vi "rio 9030 3.vi"() -> ()   [LabVIEW 2015]
uses:
  <vilib>/Platform/TimedLoop/XDataNode/timing_clust.ctl
  <vilib>/Platform/TimedLoop/XDataNode/nitl_modes.ctl
  <vilib>/Platform/TimedLoop/XDataNode/wakeup.ctl
  <vilib>/FPGAPlugInAG/cRIO-9030/niLvFpga_Open_cRIO-9030.vi
  <vilib>/rvi/interface/common/dynamic/niFpgaDynamicAddResources.vi
  <vilib>/FPGAPlugInAG/Dynamic/niLvFpga_Abort_Dynamic.vi
  <vilib>/FPGAPlugInAG/Dynamic/niLvFpga_Run_Dynamic.vi
  rio_Global.vi
  <vilib>/Utility/error.llb/Error Cluster From Error Code.vi
  <vilib>/rvi/errors/niLvFpgaAdjustHostInterfaceError.vi
  <vilib>/Analysis/Matrix/Numeric/Conversions/Array To Matrix - RA2.vi
  <vilib>/Analysis/Matrix/Numeric/Multiply/Multiply - RM,RM.vi
  <vilib>/Analysis/Matrix/Numeric/Add/Add - RM,RM.vi
  <vilib>/Analysis/baseanly.llb/Real Inverse Matrix.vi
  <vilib>/Analysis/Matrix/Numeric/Subtract/Subtract - RM,RM.vi
  <vilib>/Analysis/Matrix/Numeric/Conversions/Array To Matrix - RA.vi
  <vilib>/Analysis/Matrix/Numeric/Multiply/Multiply - R,RM.vi
  <vilib>/Analysis/Matrix/Numeric/Conversions/Matrix To Array - RM.vi
  <vilib>/rvi/interface/nirviOpenFPGA/nirviOpenFPGA.xnode
  FPGA Bitfiles/autonomous_FPGATarget4_fpga1_rudp+OsNkSQ.lvbitx
  samsung/fpga 1.vi
  <vilib>/rvi/interface/nirviMethod/nirviMethod.xnode
  <vilib>/rvi/interface/nirviReadWriteControl/nirviReadWriteControl.xnode
  <vilib>/platform/TimedLoop/XDataNode/XDataNode.xnode
  <vilib>/FPGAPlugInAG/Dynamic/niLvFpga_ReadFifo_Dynamic.vi
  <vilib>/rvi/errors/niLvFpgaMergeErrorWithErrorCode.vi
  <vilib>/Analysis/Matrix/NI_Matrix.lvlib
  <vilib>/Analysis/NI_AALBase.lvlib
  <vilib>/rvi/interface/Simulation/niFpgaSimulationCallBeginRW.vi
  NiFpgaLv.dll
  <vilib>/addons/control/pid/NI_PID_pid.lvlib
  <vilib>/ptbypt/NI_PtbyPt.lvlib
  <vilib>/Platform/TimedLoop/XDataNode/XDNodeRunTimeDep.lvlib
  <vilib>/addons/control/pid/pid.llb/PID (DBL).vi
panel:
  out "vel_ave":dbl
  out "dt vel":dbl
  out "dt":dbl
  in  "GPS on":bool=TRUE
  out "conutpos":i32
  in  "V_PID_gain":dbl[](array[numeric])=[3.0, 10.0, 4.0]
  out "FPGA":refnum<k20>
  in  "GPS Update km/h":dbl=15.0 format="%#_13g"
  out "map name":T1(ring)=enum."KAIST"
  out "con_dt":dbl
  in  "Dial":dbl(knob) min=-360.0 max=360.0 step=5.0 scale=-360.0..360.0
  out "C_yaw_rate":dbl
  in  "speed control":bool
  out "C_MCP":dbl
  out "C_APV":dbl
  out "Ref_VS":dbl
  out "XY Graph":cluster{"Y":dbl[], "Y":dbl[]}[](graph)=[{"Y"=[1.82421875, 1.8301353427767753, 1.835194070339203, 1.8394013252854347, 1.8427635002136231, 1.84528698772192, 1.8469781804084777, 1.8478434708714486, 1.8478892517089844, 1.8471219155192375, 1.84554785490036, 1.8431734624505043, 1.8400051307678222, 1.8360492524504661, 1.8313122200965881, 1.8258004263043404, 1.819520263671875, 1.8124781247973443, 1.8046804022789003, 1.796133488714695, 1.7868437767028809, 1.77681765884161, 1.7660615277290344, 1.7545817759633064, 1.742384796142578, 1.7294769808650017, 1.7158647227287291, 1.701554414331913, 1.686552448272705, 1.6708652171492577, 1.654499113559723, 1.637460530102253, 1.619755859375, 1.6013914939761162, 1.5823738265037537, 1.5627092495560646, 1.5424041557312012, 1.5214649376273155, 1.4998979878425598, 1.4777096989750862, 1.4549064636230469, 1.431494674384594, 1.4074807238578795, 1.3828710046410562, 1.3576719093322753, 1.3318898305296898, 1.3055311608314515, 1.2786022928357124, 1.251109619140625, 1.2230595323443412], "Y"=[0.0, 0.5, 1.0, 1.5, 2.0, 2.5, 3.0, 3.5, 4.0, 4.5, 5.0, 5.5, 6.0, 6.5, 7.0, 7.5, 8.0, 8.5, 9.0, 9.5, 10.0, 10.5, 11.0, 11.5, 12.0, 12.5, 13.0, 13.5, 14.0, 14.5, 15.0, 15.5, 16.0, 16.5, 17.0, 17.5, 18.0, 18.5, 19.0, 19.5, 20.0, 20.5, 21.0, 21.5, 22.0, 22.5, 23.0, 23.5, 24.0, 24.5]}, {"Y"=[-1.22265625, -1.2167396572232247, -1.211680929660797, -1.2074736747145653, -1.2041114997863769, -1.20158801227808, -1.1998968195915223, -1.1990315291285514, -1.1989857482910156, -1.1997530844807625, -1.20132714509964, -1.2037015375494957, -1.2068698692321778, -1.2108257475495339, -1.2155627799034119, -1.2210745736956596, -1.227354736328125, -1.2343968752026557, -1.2421945977210997, -1.250741511285305, -1.2600312232971191, -1.27005734115839, -1.2808134722709656, -1.2922932240366936, -1.304490203857422, -1.3173980191349983, -1.3310102772712709, -1.345320585668087, -1.360322551727295, -1.3760097828507423, -1.392375886440277, -1.409414469897747, -1.427119140625, -1.4454835060238838, -1.4645011734962463, -1.4841657504439354, -1.5044708442687988, -1.5254100623726845, -1.5469770121574402, -1.5691653010249138, -1.5919685363769531, -1.615380325615406, -1.6393942761421205, -1.6640039953589438, -1.6892030906677247, -1.7149851694703102, -1.7413438391685485, -1.7682727071642876, -1.795765380859375, -1.8238154676556588, -1.8524165749549866, -1.8815623101592065, -1.911246280670166, -1.9414620938897134, -1.972203357219696, -2.003463678061962, -2.0352366638183597, -2.0675159218907355, -2.1002950596809384, -2.1335676845908162, -2.167327404022217, -2.2015678253769875, -2.2362825560569766, -2.2714652034640315, -2.307109375, -2.3432086780667305, -2.3797567200660703, -2.4167471083998677, -2.4541734504699706, -2.4920293536782263, -2.530308425426483, -2.5690042731165885, -2.6081105041503907, -2.647620725929737, -2.687528545856476, -2.7278275713324547, -2.7685114097595216, -2.809573668539524, -2.8510079550743104, -2.892807876765728, -2.934967041015625, -2.977479055225849, -3.020337526798248, -3.0635360631346704, -3.107068271636963, -3.150927759706974, -3.1951081347465515, -3.2396030041575434, -3.284405975341797, -3.3295106557011604, -3.3749106526374817, -3.4205995735526087, -3.466571025848389, -3.51281861692667, -3.5593359541893004], "Y"=[0.0, 0.5, 1.0, 1.5, 2.0, 2.5, 3.0, 3.5, 4.0, 4.5, 5.0, 5.5, 6.0, 6.5, 7.0, 7.5, 8.0, 8.5, 9.0, 9.5, 10.0, 10.5, 11.0, 11.5, 12.0, 12.5, 13.0, 13.5, 14.0, 14.5, 15.0, 15.5, 16.0, 16.5, 17.0, 17.5, 18.0, 18.5, 19.0, 19.5, 20.0, 20.5, 21.0, 21.5, 22.0, 22.5, 23.0, 23.5, 24.0, 24.5, 25.0, 25.5, 26.0, 26.5, 27.0, 27.5, 28.0, 28.5, 29.0, 29.5, 30.0, 30.5, 31.0, 31.5, 32.0, 32.5, 33.0, 33.5, 34.0, 34.5, 35.0, 35.5, 36.0, 36.5, 37.0, 37.5, 38.0, 38.5, 39.0, 39.5, 40.0, 40.5, 41.0, 41.5, 42.0, 42.5, 43.0, 43.5, 44.0, 44.5, 45.0, 45.5, 46.0, 46.5, 47.0]}, {"Y"=[-0.94, 0.94, 0.94, -0.94, -0.94], "Y"=[-3.2, -3.2, 1.5, 1.5, -3.2]}, {"Y"=[1.984375, 1.978057861328125, 1.9718017578125, 1.965606689453125, 1.95947265625], "Y"=[0.0, 0.5, 1.0, 1.5, 2.0]}, {"Y"=[-5.28125, -5.267578125, -5.25390625, -5.240234375, -5.2265625], "Y"=[0.0, 0.5, 1.0, 1.5, 2.0]}]
  in  "Manual Steering torque":dbl(slide) min=-0.9 max=0.9 step=0.01 scale=-0.9..0.9
  out "Mobileye_time 50":u32
  out "H_GPS":dbl
  out "vgain":dbl=1.0
  out "vcount":u64=1
  out "hbias":dbl
  out "hcount":u64=1
  out "get heading":bool
  out "get position":bool
  out "heading error":dbl
  out "h_gps":dbl
  out "pos error":dbl
  out "POS init":bool
  out "Heading":dbl
  out "pos":dbl[](array[numeric])
  in  "GPS init":bool=TRUE
  out "pos_gps":dbl[](array[numeric]) format="%#_19f"
  out "dt yaw":dbl
  out "ecef ref":dbl[](array[numeric])
  in  "Velocity input":bool
  in  "Manual Speed":dbl=20.0
  in  "Steer input":bool=TRUE
  out "Run":bool
  out "Auto":bool
  out "E - STOP":bool
  out "Con_time 10":i32
  out "VS_CAN":dbl
  out "CAN_time 10":u32
  out "gps1":refnum<visa-resource-name>
  out "x_view":dbl[](array[numeric])=[0.0, 0.5, 1.0, 1.5, 2.0, 2.5, 3.0, 3.5, 4.0, 4.5, 5.0, 5.5, 6.0, 6.5, 7.0, 7.5, 8.0, 8.5, 9.0, 9.5, 10.0, 10.5, 11.0, 11.5, 12.0, 12.5, 13.0, 13.5, 14.0, 14.5, 15.0, 15.5, 16.0, 16.5, 17.0, 17.5, 18.0, 18.5, 19.0, 19.5, 20.0, 20.5, 21.0, 21.5, 22.0, 22.5, 23.0, 23.5, 24.0, 24.5, 25.0, 25.5, 26.0, 26.5, 27.0, 27.5, 28.0, 28.5, 29.0, 29.5, 30.0, 30.5, 31.0, 31.5, 32.0, 32.5, 33.0, 33.5, 34.0, 34.5, 35.0, 35.5, 36.0, 36.5, 37.0, 37.5, 38.0, 38.5, 39.0, 39.5, 40.0, 40.5, 41.0, 41.5, 42.0, 42.5, 43.0, 43.5, 44.0, 44.5, 45.0, 45.5, 46.0, 46.5, 47.0, 47.5, 48.0, 48.5, 49.0, 49.5, 50.0, 50.5, 51.0, 51.5, 52.0, 52.5, 53.0, 53.5, 54.0, 54.5, 55.0, 55.5, 56.0, 56.5, 57.0, 57.5, 58.0, 58.5, 59.0, 59.5, 60.0, 60.5, 61.0, 61.5, 62.0, 62.5, 63.0, 63.5, 64.0, 64.5, 65.0, 65.5, 66.0, 66.5, 67.0, 67.5, 68.0, 68.5, 69.0, 69.5, 70.0, 70.5, 71.0, 71.5, 72.0, 72.5, 73.0, 73.5, 74.0, 74.5, 75.0, 75.5, 76.0, 76.5, 77.0, 77.5, 78.0, 78.5, 79.0, 79.5, 80.0, 80.5, 81.0, 81.5, 82.0, 82.5, 83.0, 83.5, 84.0, 84.5, 85.0, 85.5, 86.0, 86.5, 87.0, 87.5, 88.0, 88.5, 89.0, 89.5, 90.0, 90.5, 91.0, 91.5, 92.0, 92.5, 93.0, 93.5, 94.0, 94.5, 95.0, 95.5, 96.0, 96.5, 97.0, 97.5, 98.0, 98.5, 99.0, 99.5, 100.0, 100.5, 101.0, 101.5, 102.0, 102.5, 103.0, 103.5, 104.0, 104.5, 105.0, 105.5, 106.0, 106.5, 107.0, 107.5, 108.0, 108.5, 109.0, 109.5, 110.0, 110.5, 111.0, 111.5, 112.0, 112.5, 113.0, 113.5, 114.0, 114.5, 115.0, 115.5, 116.0, 116.5, 117.0, 117.5, 118.0, 118.5, 119.0, 119.5, 120.0, 120.5, 121.0, 121.5, 122.0, 122.5, 123.0, 123.5, 124.0, 124.5, 125.0, 125.5, 126.0, 126.5, 127.0, 127.5, 128.0]
  out "T init":i32
  out "T out":i32
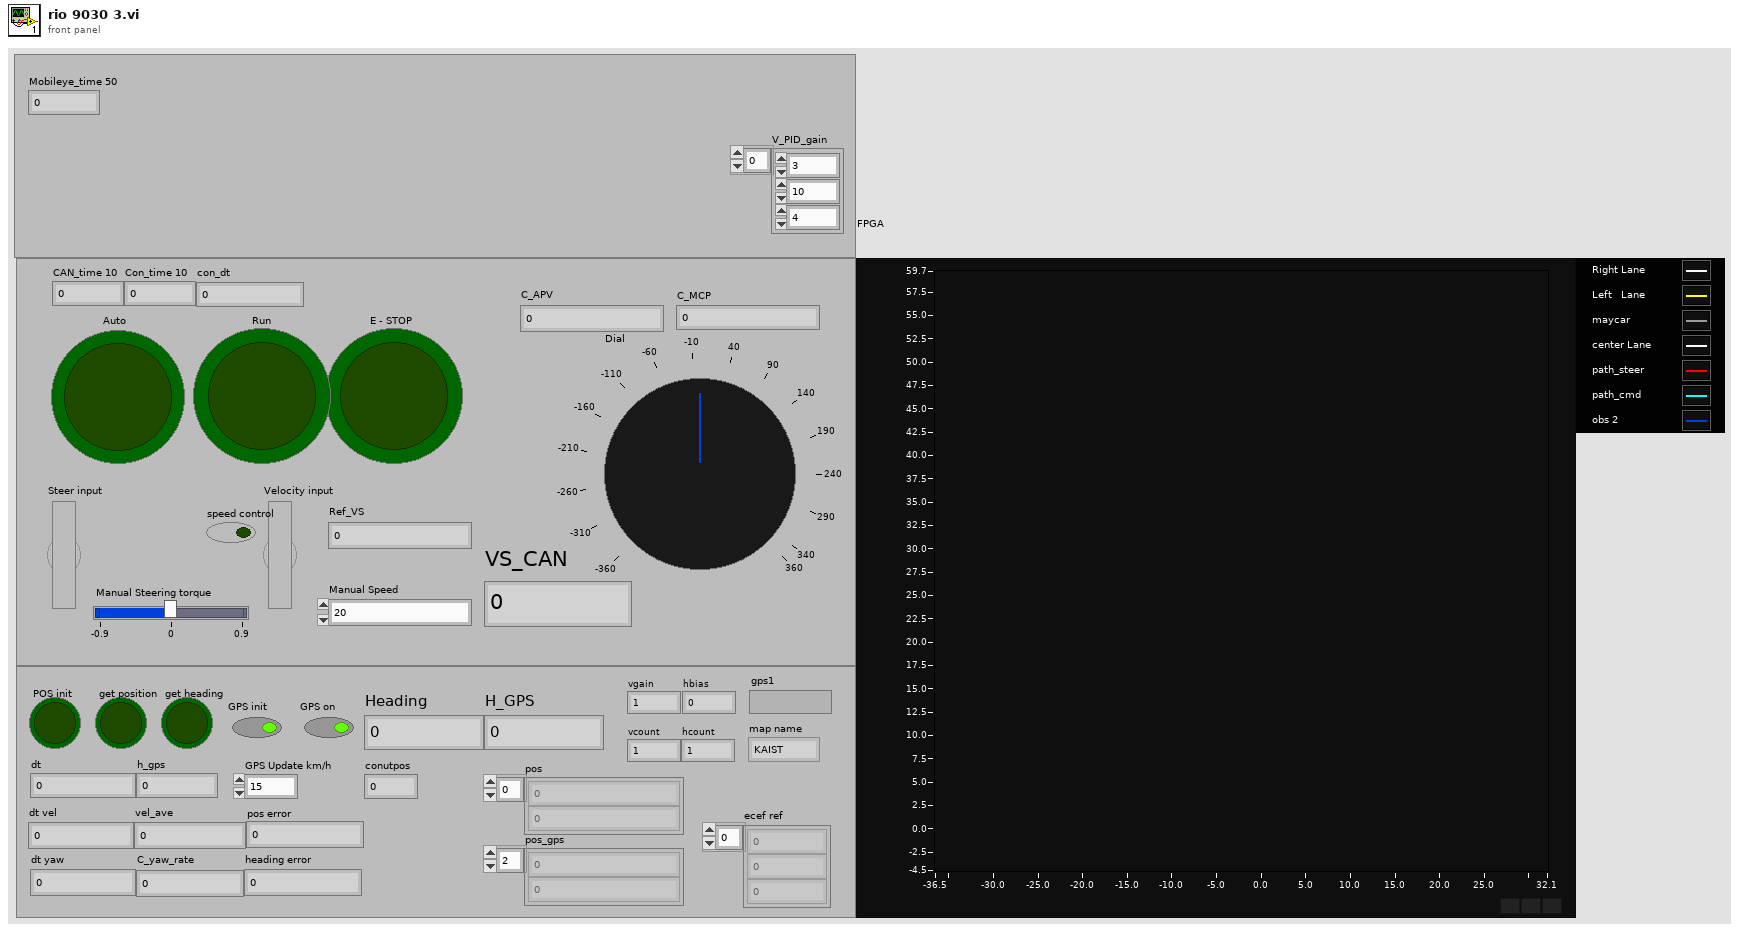
[diagram p1: front panel]
types:
  T1 = enum32{"Namyang", "Hyundai", "KAIST", "Ajou", "Munji", "Airforce", "Car", "KATRI", "Samsung", "Coex", "Gwangnaru", "Inje", "sinjin", "NAVER"}
  T2 = cluster{"identifier":u32, "timestamp":timestamp, "payload":u8[]}
  T3 = cluster{"timestamp high":u32, "timestamp low":u32, "identifier":u32, "type":enum8{"Data Frame", "Remote Frame", "(reserved)", "(reserved) ", "(reserved)  ", "(reserved)   ", "Bus Error", "Transceiver Fault"}, "info A":u8, "info B":u8, "data length":u8, "data":u8[]}
  T4 = cluster{"connection ID":refnum<k16>, "net address":u32, "port":u16}
  T5 = cluster{"hash":i64, "sys time":i64, "size":i32, "data":u8[]}
  T6 = cluster{"hash":i64, "sys time":i64, "time":dbl, "yaw_rate":dbl, "mdps torque":dbl, "mdps str_ang":dbl, "VS_CAN":dbl, "lat_accel":dbl, "mcp":dbl, "accel pedal value":dbl, "tps":dbl, "odometer":dbl, "battery voltage":dbl, "WHL_SPD_RR":dbl, "WHL_SPD_RL":dbl, "WHL_SPD_FR":dbl, "WHL_SPD_FL":dbl}
  T7 = cluster{"proportional gain (Kc)":dbl, "integral time (Ti, min)":dbl, "derivative time (Td, min)":dbl}
  T8 = cluster{"hash":i64, "sys time":i64, "ref_vel":dbl, "ref_steer":dbl, "alert":u8}
  T9 = cluster{"hash":i64, "sys time":i64, "ref_vel":dbl, "ref_steer":dbl}
  T10 = cluster{"hash":i64, "sys time":i64, "Auto":bool, "Run":bool, "Solenoid":bool, "T lim":bool, "brk_enc":u8, "B PWM":u16, "T PWM":u16, "ref_vel":dbl, "ref_bkr_enc":dbl, "ref_apv":dbl, "ref_steer":dbl, "net address":u32}
  T11 = enum32{"Namyang", "Hyundai", "KAIST", "Ajou", "Munji", "Airforce", "Car", "KATRI", "Samsung", "Coex", "Gwangnaru", "Inje", "sinjin"}
  T12 = typedef "XDNodeRunTimeDep.lvlib/timing_clust.ctl" = cluster{"Expected End [f-1]":u64, "Actual End [f-1]":u64, "Finished Late? [f-1]":bool, "Expected End [i-1]":u64, "Actual End [i-1]":u64, "Finished Late? [i-1]":bool, "Expected Start [i]":u64, "Actual Start [i]":u64, "Expected Start [f]":u64, "Actual Start [f]":u64, "Source Name":string, "Structure Name":string, "Period":i64, "Deadline":i64, "Offset":i64, "Start":i64, "Priority":i32, "Timeout":i32, "Mode":T13, "Wakeup Reason":T14, "Error":errorcluster, "Source Type":string, "Secondary Source Type":string, "Global End Time":u64, "Global Start Time":u64, "Frame Duration":u64, "Iteration Duration":u64, "Assigned CPU":i32, "I/O Scan Engine Mode":u32}
  T13 = typedef "XDNodeRunTimeDep.lvlib/nitl_modes.ctl" = enum32{"No Change", "Process missed periods, maintain original phase", "Discard missed periods, maintain original phase", "Process missed periods, ignore original phase", "Discard missed periods, ignore original phase"}
  T14 = typedef "XDNodeRunTimeDep.lvlib/wakeup.ctl" = enum32{"Normal", "Aborted", "Asynchronous wakeup", "Timing source error", "Timed loop error", "Timeout"}
  T15 = cluster{"hash":i64, "sys time":i64, "time":dbl, "x":dbl, "y":dbl, "h":dbl, "numSV":i32, "postype":i32, "lag":i32, "hordev":dbl, "lat":dbl, "lon":dbl, "hgt":dbl, "map_idx":i32}
  T16 = cluster{"output[0]":dbl, "output[1]":dbl, "output[2]":dbl, "output[3]":dbl, "output[4]":dbl, "output[5]":dbl, "output[6]":dbl, "output[7]":dbl, "output[8]":dbl, "output[9]":dbl, "output[10]":dbl, "output[11]":dbl, "output[12]":dbl, "output[13]":dbl, "output[14]":dbl}
  T17 = cluster{"hash":i64, "sys time":i64, "time":dbl, "speed":dbl, "heading":dbl, "lat":dbl, "lon":dbl}
  T18 = cluster{"output[0]":dbl, "output[1]":dbl, "output[2]":dbl, "output[3]":dbl, "output[4]":dbl, "output[5]":dbl, "output[6]":dbl}
  T19 = typedef "NI_Matrix.lvlib/RealMatrix.ctl" = dbl[][]
  T20 = cluster{"hash":i64, "sys time":i64, "dt":dbl, "x":dbl, "y":dbl, "speed":dbl, "heading":dbl, "yaw_rate":dbl}
  T21 = cluster{"Real 2D Array[0]":dbl, "Real 2D Array[1]":dbl, "Real 2D Array[2]":dbl, "Real 2D Array[3]":dbl, "Real 2D Array[4]":dbl}
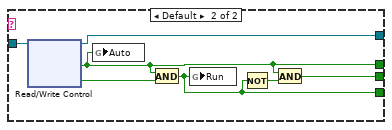
[diagram p3: hidden frame]
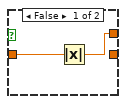
[diagram p7: hidden frame]
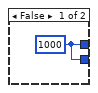
[diagram p8: hidden frame]
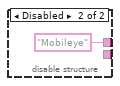
[diagram p9: hidden frame]
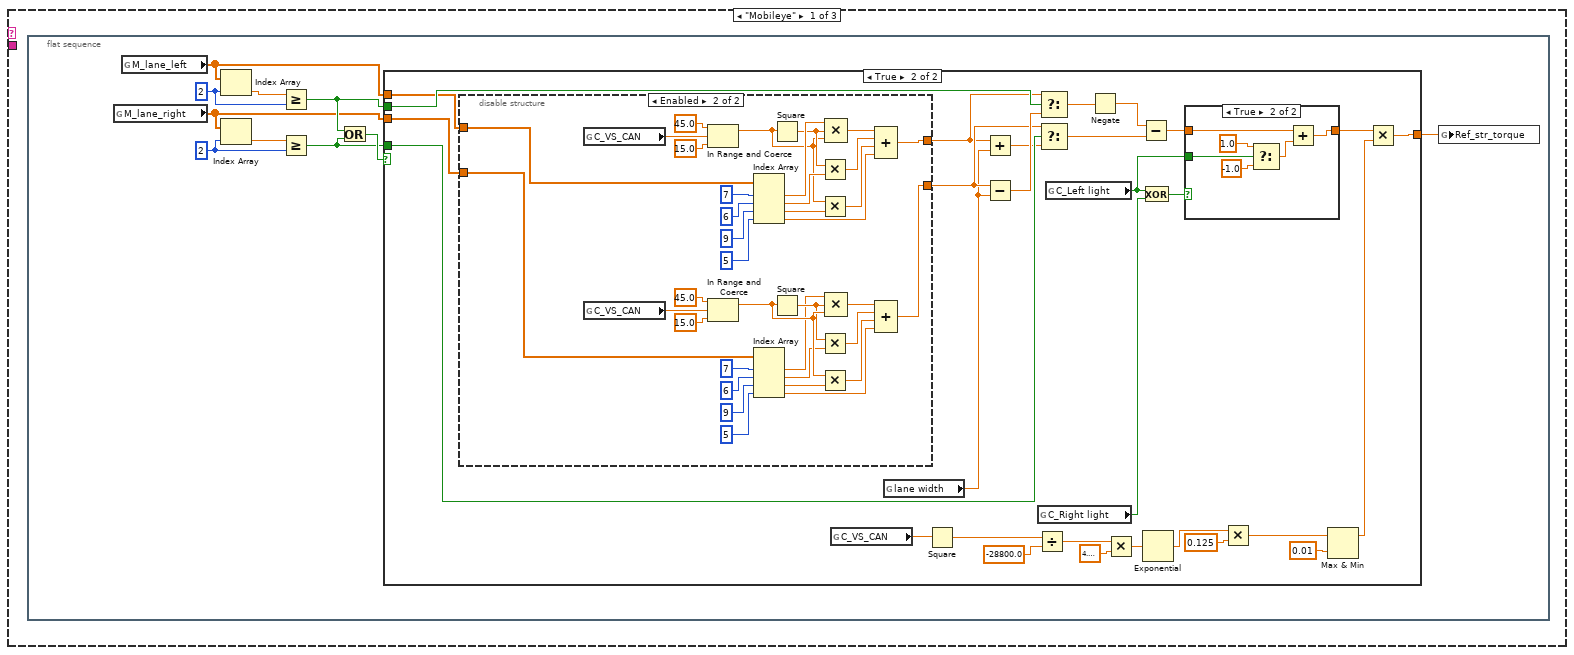
[diagram p10: hidden frame]
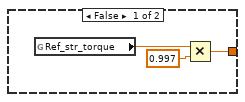
[diagram p11: hidden frame]
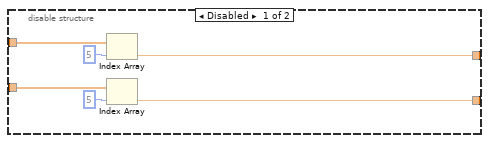
[diagram p12: hidden frame]
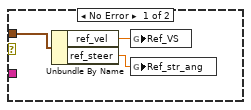
[diagram p14: hidden frame]
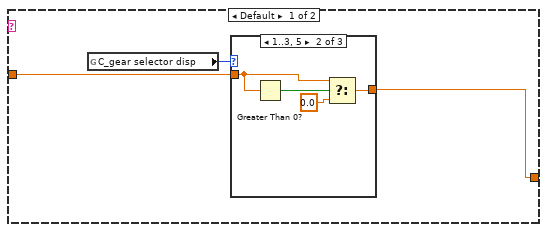
[diagram p17: hidden frame]
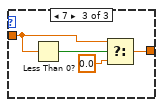
[diagram p19: hidden frame]
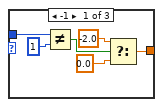
[diagram p20: hidden frame]
diagram:
  n1 = while {
    stop <- FALSE stop-if-true
    n2 = flat-sequence {
      tunnel: [w8] -> w2
      tunnel: w2 -> [w38]
      frame #0 {
        n3 = Wait Until Next ms Multiple(millisecond multiple=u32 10) -> ()  [unwired: 1 out]
      }
      frame #1 {
        n4 = global read "rio_Global.vi" "Car_name"() -> (w5:string)
        n5 = local read "FPGA"() -> (w10:refnum<k20>)
        n6 = case shown="\"Prius\", \"Santafe\"" w5 {
          tunnel: w10 -> [w13 w20]
          tunnel: [_ w18] -> w9
          tunnel: [w13 w16] -> w8
          tunnel: [w12 w15] -> w7
          tunnel: [w11 w14] -> w6
          frame "Prius", "Santafe" {
            n7 = global read "rio_Global.vi" "Auto"() -> (w12:bool)
            n8 = global read "rio_Global.vi" "Run"() -> (w11:bool)
          }
          frame Default {
            n9 = xnode "Read/Write Control"("FPGA VI Reference In"=w20) -> ("FPGA VI Reference Out"=w16:refnum<k20>, "Auto"=w15:bool, "Run"=w19:bool)  [unwired: 1 in, 1 out]
            n10 = global write "rio_Global.vi" "Auto"(w15) -> ()
            n11 = And(x=w15, y=w19) -> (x .and. y?=w14:bool)
            n12 = global write "rio_Global.vi" "Run"(w14) -> ()
            n13 = Not(x=w14) -> (.not. x?=w17:bool)
            n14 = And(x=w15, y=w17) -> (x .and. y?=w18:bool)
          }
        }
        "E - STOP" <- w9
        "Auto" <- w7
        "Run" <- w6
      }
      frame #2 {
        w30 = fxp<+/-,20,5> 0.0 ("Mod3/AO3")
        n15 = global read "rio_Global.vi" "Car_name"() -> (w26:string)
        n16 = global read "rio_Global.vi" "Auto"() -> (w24:bool)
        n17 = case shown="\"Prius\"" w26 {
          tunnel: [_ w42] -> w28
          tunnel: [_ w41] -> w21
          frame Default {
          }
          frame "Prius" {
            n18 = global read "rio_Global.vi" "Shift control"() -> (w43:dbl)
            n19 = global read "rio_Global.vi" "C_VS_CAN"() -> (w45:dbl)
            n20 = Not Equal To 0?(x=w43) -> (x != 0?=w40:bool)
            n21 = Equal To 0?(x=w45) -> (x = 0?=w46:bool)
            n22 = global read "rio_Global.vi" "Auto"() -> (w39:bool)
            n23 = Compound Arithmetic op=AND(w40, w46, w39) -> (w44:bool)
            n24 = case shown="True" w44 {
              selector: w44 -> [_ w47]
              tunnel: w43 -> [_ w48]
              tunnel: [_ w48] -> w42
              tunnel: [_ w47] -> w41
              frame False {
              }
              frame True {
              }
            }
          }
        }
        n25 = global read "rio_Global.vi" "Auto"() -> (w29:bool)
        n26 = And(x="speed control", y=w24) -> (x .and. y?=w23:bool)
        n27 = case shown="True" w23 {
          tunnel: [w56 w69] -> w37
          tunnel: [w56 w68] -> w36
          tunnel: [_ w63] -> w35
          frame False {
            w56 = u16 1000
          }
          frame True {
            n28 = global read "rio_Global.vi" "PWM Brake"() -> (w62:dbl)
            n29 = global read "rio_Global.vi" "PWM GAS"() -> (w71:dbl)
            n30 = Round To Nearest(number=w71) -> (nearest integer value=w66:dbl)
            n31 = Round To Nearest(number=w62) -> (nearest integer value=w61:dbl)
            n32 = global read "rio_Global.vi" "Run"() -> (w59:bool)
            n33 = global read "rio_Global.vi" "Run"() -> (w60:bool)
            n34 = global read "rio_Global.vi" "Solenoid"() -> (w65:bool)
            n35 = Select(t=w66, s=w59, f=1000.0) -> (s? t:f=w64:dbl)
            n36 = Select(t=w61, s=w60, f=1900.0 ("t")) -> (s? t:f=w57:dbl)
            n37 = global read "rio_Global.vi" "Run"() -> (w58:bool)
            n38 = To Unsigned Word Integer(number=w64) -> (unsigned 16bit integer=w69:u16)
            n39 = To Unsigned Word Integer(number=w57) -> (unsigned 16bit integer=w68:u16)
            n40 = Select(t=w65, s=w58, f=w58) -> (s? t:f=w63:bool)
          }
        }
        n41 = case shown="True" w29 {
          tunnel: [_ w50] -> w34
          tunnel: [_ w49] -> w33
          frame False {
          }
          frame True {
            n42 = global read "rio_Global.vi" "steering torque"() -> (w51:dbl)
            n43 = Greater Than 0?(x=w51) -> (x > 0?=w52:bool)
            n44 = case shown="True" w52 {
              tunnel: w51 -> [w54 w55]
              tunnel: [w53 _] -> w50
              tunnel: [_ w55] -> w49
              frame False {
                n45 = Absolute Value(x=w54) -> (abs(x)=w53:dbl)
              }
              frame True {
              }
            }
          }
        }
        n46 = To Fixed-Point(fixed-point type=w30, number=w34) -> (fixed-point=w32:fxp<+/-,20,5>)
        n47 = To Fixed-Point(fixed-point type=w30, number=w33) -> (fixed-point=w31:fxp<+/-,20,5>)
        n48 = To Fixed-Point(fixed-point type=fxp<+/-,20,5> 0.0 ("Mod3/AO3"), number=w28) -> (fixed-point=w22:fxp<+/-,20,5>)
        n49 = xnode "Read/Write Control"("FPGA VI Reference In"=w38, "Solenoid"=w35, "PWM Gas"=w37, "PWM Brake"=w36, "Mod3/AO0"=w32, "Mod3/AO1"=w31, "Mod3/AO3"=w22, "Mod1/DIO3"=w21) -> ()  [unwired: 1 in, 2 out]
      }
    }
  }
  n50 = flat-sequence {
    frame #0 {
      w73 = u16 7668 ("port")
      w82 = u16 7667 ("port")
      n51 = disable-structure shown="Enabled" {
        frame Disabled {
        }
        frame Enabled {
          w90 = "Prius" ("Car_name")
          w96 = 0.0 ("Ref_str_ang")
          w97 = 1000.0 ("PWM GAS")
          w95 = FALSE ("Auto SW")
          n52 = global write "rio_Global.vi" "Shift control"(0.0 ("Shift control")) -> ()
          n53 = global write "rio_Global.vi" "steering torque"(0.0 ("steering")) -> ()
          n54 = global write "rio_Global.vi" "Solenoid"(FALSE ("CAN A 1")) -> ()
          n55 = global write "rio_Global.vi" "Ref_VS"(w96) -> ()
          n56 = global write "rio_Global.vi" "Ref_str_ang"(w96) -> ()
          n57 = global write "rio_Global.vi" "PWM GAS"(w97) -> ()
          n58 = global write "rio_Global.vi" "PWM Brake"(w97) -> ()
          n59 = global write "rio_Global.vi" "Auto"(w95) -> ()
          n60 = global write "rio_Global.vi" "Car_name"(w90) -> ()
          n61 = call "car_spec.vi"("Car_name"=w90) -> ("turn radius"=w94:dbl, "wheel base"=w93:dbl, "ratio"=w92:dbl, "overall width"=w91:dbl)  [unwired: 5 in, 2 out]
          n62 = global write "rio_Global.vi" "Auto SW"(w95) -> ()
          n63 = global write "rio_Global.vi" "ratio"(w92) -> ()
          n64 = global write "rio_Global.vi" "overall width"(w91) -> ()
          n65 = global write "rio_Global.vi" "wheel base"(w93) -> ()
          n66 = global write "rio_Global.vi" "turn radius"(w94) -> ()
        }
      }
      n67 = xnode "Open FPGA VI Reference"() -> ("FPGA VI Reference Out"=w84:refnum<k20>, "error out"=w85:errorcluster)  [unwired: 2 in]
      n68 = global read "rio_Global.vi" "LCM PC"() -> (w77:T4)
      n69 = Decrement(x=w82) -> (x-1=w83:u16)
      n70 = UDP Open(11:w73) -> (port=w75:refnum<k16>)  [unwired: 4 in, 2 out]
      n71 = xnode "Invoke Method"("FPGA VI Reference In"=w84, "error in"=w85) -> ("FPGA VI Reference Out"=w86:refnum<k20>, "error out"=w87:errorcluster)
      n72 = Bundle By Name(cluster=w77, "port"=w73, "connection ID"=w75, "net address"=u32 0) -> (w76:T4)
      n73 = UDP Open(11:w83) -> (port=w80:refnum<k16>)  [unwired: 4 in, 2 out]
      n74 = xnode "Invoke Method"("FPGA VI Reference In"=w86, "error in"=w87, "Wait Until Done (F)"=FALSE) -> ("FPGA VI Reference Out"=→"FPGA":refnum<k20>)  [unwired: 1 out]
      n75 = global read "rio_Global.vi" "LCM"() -> (w78:T4)
      n76 = Bundle By Name(cluster=w78, "port"=w82, "connection ID"=w80, "net address"=u32 4294967295) -> (w79:T4)
      n77 = global write "rio_Global.vi" "LCM PC"(w76) -> ()
      n78 = global write "rio_Global.vi" "LCM"(w79) -> ()
    }
    frame #1 {
      n79 = flat-sequence {
        tunnel: [w102] -> w101
        tunnel: w101 -> [w109]
        frame #0 {
          n80 = local read "FPGA"() -> (w103:refnum<k20>)
          n81 = xnode "Invoke Method"("FPGA VI Reference In"=w103, "Number of Elements"=u32 0, "Timeout (ms)"=0) -> ("FPGA VI Reference Out"=w105:refnum<k20>, "Elements Remaining"=w106:u32)  [unwired: 1 in, 2 out]
          n82 = xnode "Invoke Method"("FPGA VI Reference In"=w105, "Number of Elements"=w106, "Timeout (ms)"=0) -> ("FPGA VI Reference Out"=w102:refnum<k20>)  [unwired: 1 in, 3 out]
        }
        frame #1 {
          n83 = while {
            tunnel: w109 -> [w110]
            stop <- FALSE stop-if-true
            n84 = flat-sequence {
              tunnel: [w113] -> w111
              tunnel: w110 -> [w113]
              tunnel: w111 -> [w120]
              frame #0 {
                n85 = Wait Until Next ms Multiple(millisecond multiple=u32 50) -> (millisecond timer value=w115:u32)
                n86 = feedback #1(w115) -> (w116:u32)
                n87 = feedback-in #1(w115) -> ()
                n88 = Subtract(x=w115, y=w116) -> (x-y=→"Mobileye_time 50":u32)
              }
              frame #1 {
                n89 = while {
                  tunnel: w120 -> [w166]
                  tunnel: [w163] -> w119 mode=indexing
                  stop <- w161 stop-if-true
                  n90 = xnode "Invoke Method"("FPGA VI Reference In"=w166, "Number of Elements"=u32 16, "Timeout (ms)"=0) -> ("FPGA VI Reference Out"=w162:refnum<k20>, "Data"=w163:u8[], "Elements Remaining"=w160:u32)  [unwired: 1 in, 1 out]
                  n91 = Equal To 0?(x=w160) -> (x = 0?=w161:bool)
                  n92 = Quotient & Remainder(x=w160, y=u32 16) -> (x-y*floor(x/y)=w158:u32)  [unwired: 1 out]
                  n93 = case shown="1, Default" w158 {
                    selector: w158 -> [w169 _]
                    tunnel: w162 -> [w168 _]
                    frame 1, Default {
                      n94 = xnode "Invoke Method"("FPGA VI Reference In"=w168, "Number of Elements"=w169, "Timeout (ms)"=0) -> ()  [unwired: 1 in, 4 out]
                    }
                    frame 0 {
                    }
                  }
                }
                n95 = Empty Array?(array=w119) -> (empty?=w118:bool)
                n96 = case shown="False" w118 {
                  tunnel: w119 -> [w122 _]
                  frame False {
                    n97 = flat-sequence {
                      tunnel: w122 -> [w123]
                      tunnel: [w123] -> w121
                      tunnel: w121 -> [w142]
                      frame #0 {
                        n98 = for {
                          tunnel: w123 -> [w133] mode=indexing
                          w136 = 4 ("length")
                          w134 = 8 ("index")
                          n99 = Delete From Array(array=w133, length=w134, index=w134) -> (deleted portion=w124:u8[], array with subset deleted=w135:u8[])
                          n100 = Delete From Array(array=w135, length=w136, index=w136) -> (deleted portion=w140:u8[], array with subset deleted=w137:u8[])
                          n101 = Type Cast(type=u32 0, x=w137) -> (*(type *) &x=w125:u32)
                          n102 = Type Cast(type=u32 0, x=w140) -> (*(type *) &x=w126:u32)
                          n103 = Multiply(x=w126, y=1e-07) -> (x*y=w131:dbl)
                          n104 = To Time Stamp(1:w131) -> (0:w129:timestamp)
                          n105 = Bundle By Name(cluster=T2 {"identifier"=0, "timestamp"=timestamp(0 s since 1904-01-01), "payload"=[]} ("can cluster"), "identifier"=w125, "payload"=w124, "timestamp"=w129) -> (w127:T2)
                          n106 = call "mobileye_decoder.vi"("can cluster"=w127, "name"="Mobileye560") -> ()  [unwired: 10 in]
                        }
                      }
                      frame #1 {
                        n107 = Array Size(array=w142) -> (size(s)=w143:i32[])
                        n108 = Multiply Array Elements(1:w143) -> (0:w152:i32)
                        n109 = Get Date/Time In Seconds() -> (seconds since 1Jan1904=w148:timestamp)
                        n110 = To Double Precision Float(number=w148) -> (double precision float=w149:dbl)
                        n111 = Reshape Array(w142, w152) -> (w153:u8[])
                        n112 = global read "rio_Global.vi" "LCM_CAN_RAW_SNAP"() -> (w146:T5)
                        n113 = Unbundle By Name(w146) -> ("hash"=w151:i64)
                        n114 = Multiply(x=w149, y=1000000.0) -> (x*y=w147:dbl)
                        n115 = To Quad Integer(1:w147) -> (0:w144:i64)
                        n116 = call "hash.vi"("input"=w151) -> ("output"=w145:i64)  [unwired: 10 in]
                        n117 = Bundle(cluster=w146, "hash"=w145, "sys time"=w144, "size"=w152, "data"=w153) -> (w155:T5)
                        n118 = Flatten To String(anything=w155, prepend array or string size? (T)=FALSE) -> (data string=w157:string)  [unwired: 2 in, 2 out]
                        n119 = global read "rio_Global.vi" "LCM"() -> (w156:T4)
                        n120 = call "LCM_send.vi"("DATA"=w157, "ID"="Mobileye560" ("name"), "LCM"=w156) -> ()  [unwired: 7 in, 2 out]
                      }
                    }
                  }
                  frame True {
                  }
                }
              }
            }
          }
        }
      }
      n121 = flat-sequence {
        tunnel: [w170] -> w100
        tunnel: w100 -> [w211]
        frame #0 {
          n122 = global read "rio_Global.vi" "Car_name"() -> (w172:string)
          n123 = local read "FPGA"() -> (w171:refnum<k20>)
          n124 = case shown="Default" w172 {
            tunnel: w171 -> [w173 w179]
            tunnel: [w173 w174] -> w170
            frame "Prius" {
            }
            frame Default {
              n125 = xnode "Invoke Method"("FPGA VI Reference In"=w179, "Number of Elements"=u32 0, "Timeout (ms)"=0) -> ("FPGA VI Reference Out"=w181:refnum<k20>, "Elements Remaining"=w180:u32)  [unwired: 1 in, 2 out]
              n126 = xnode "Invoke Method"("FPGA VI Reference In"=w181, "Number of Elements"=w180, "Timeout (ms)"=0) -> ("FPGA VI Reference Out"=w177:refnum<k20>)  [unwired: 1 in, 3 out]
              n127 = flat-sequence {
                tunnel: [w192] -> w178
                tunnel: w177 -> [w192]
                frame #0 {
                  n128 = Wait (ms)(milliseconds to wait=u32 100) -> ()  [unwired: 1 out]
                }
              }
              n129 = xnode "Read/Write Control"("FPGA VI Reference In"=w178, "send can 1"=TRUE) -> ("FPGA VI Reference Out"=w187:refnum<k20>)  [unwired: 1 in, 1 out]
              n130 = for {
                N: 100 -> [_]
                tunnel: w187 -> [w195]
                tunnel: [w197] -> w175
                i -> [w194]
                n131 = Split Number(x=u16 65535 ("y")) -> (hi(x)=w206:u8, lo(x)=w205:u8)
                n132 = To Unsigned Byte Integer(number=w194) -> (unsigned 8bit integer=w193:u8)
                n133 = Build Array(u8 0 ("Con steer status"), w205, w206, u8 0 ("element"), w193, u8 0 ("element"), u8 0 ("element")) -> (w200:u8[])
                n134 = Add Array Elements(numeric array=w200) -> (sum=w201:u8)
                n135 = Build Array (concatenate)(w200, w201) -> (w198:u8[])
                n136 = Bundle By Name(cluster=T3 {"timestamp high"=0, "timestamp low"=0, "identifier"=0, "type"=enum."Data Frame", "info A"=0, "info B"=0, "data length"=8, "data"=[0, 0, 0, 0, 0, 0, 0, 0]} ("Mod4/CAN1 input"), "identifier"=u32 912, "data"=w198, "data length"=u8 8) -> (w207:T3)
                n137 = xnode "Read/Write Control"("FPGA VI Reference In"=w195, "Mod2/CAN1 input"=w207) -> ("FPGA VI Reference Out"=w197:refnum<k20>)  [unwired: 1 in, 1 out]
              }
              n138 = flat-sequence {
                tunnel: [w190] -> w176
                tunnel: w175 -> [w190]
                frame #0 {
                  n139 = Wait (ms)(milliseconds to wait=u32 100) -> ()  [unwired: 1 out]
                }
              }
              n140 = xnode "Read/Write Control"("FPGA VI Reference In"=w176, "send can 1"=FALSE) -> ("FPGA VI Reference Out"=w174:refnum<k20>)  [unwired: 1 in, 1 out]
            }
          }
        }
        frame #1 {
          n141 = while {
            tunnel: w211 -> [w212]
            stop <- FALSE stop-if-true
            n142 = flat-sequence {
              tunnel: [w215] -> w213
              tunnel: w212 -> [w215]
              tunnel: w213 -> [w222]
              frame #0 {
                n143 = Wait Until Next ms Multiple(millisecond multiple=u32 10) -> (millisecond timer value=w218:u32)
                n144 = feedback #2(w218) -> (w217:u32)
                n145 = feedback-in #2(w218) -> ()
                n146 = Subtract(x=w218, y=w217) -> (x-y=→"CAN_time 10":u32)
              }
              frame #1 {
                n147 = while {
                  tunnel: w222 -> [w284]
                  tunnel: [w281] -> w221 mode=indexing
                  stop <- w280 stop-if-true
                  n148 = xnode "Invoke Method"("FPGA VI Reference In"=w284, "Number of Elements"=u32 16, "Timeout (ms)"=0) -> ("FPGA VI Reference Out"=w279:refnum<k20>, "Data"=w281:u8[], "Elements Remaining"=w276:u32)  [unwired: 1 in, 1 out]
                  n149 = Equal To 0?(x=w276) -> (x = 0?=w280:bool)
                  n150 = Quotient & Remainder(x=w276, y=u32 16) -> (x-y*floor(x/y)=w277:u32)  [unwired: 1 out]
                  n151 = case shown="1, Default" w277 {
                    selector: w277 -> [w287 _]
                    tunnel: w279 -> [w286 _]
                    frame 1, Default {
                      n152 = xnode "Invoke Method"("FPGA VI Reference In"=w286, "Number of Elements"=w287, "Timeout (ms)"=0) -> ()  [unwired: 1 in, 4 out]
                    }
                    frame 0 {
                    }
                  }
                }
                n153 = Empty Array?(array=w221) -> (empty?=w220:bool)
                n154 = case shown="False" w220 {
                  tunnel: w221 -> [w225 _]
                  frame False {
                    n155 = flat-sequence {
                      tunnel: w225 -> [w226]
                      tunnel: [w226] -> w224
                      tunnel: w224 -> [w259]
                      tunnel: [w244] -> w223
                      tunnel: w223 -> [w271]
                      frame #0 {
                        n156 = for {
                          tunnel: w226 -> [w236] mode=indexing
                          w239 = 4 ("length")
                          w237 = 8 ("index")
                          n157 = Delete From Array(array=w236, length=w237, index=w237) -> (deleted portion=w228:u8[], array with subset deleted=w238:u8[])
                          n158 = Delete From Array(array=w238, length=w239, index=w239) -> (deleted portion=w243:u8[], array with subset deleted=w240:u8[])
                          n159 = Type Cast(type=u32 0, x=w240) -> (*(type *) &x=w229:u32)
                          n160 = Type Cast(type=u32 0, x=w243) -> (*(type *) &x=w230:u32)
                          n161 = Multiply(x=w230, y=1e-07) -> (x*y=w233:dbl)
                          n162 = To Time Stamp(1:w233) -> (0:w232:timestamp)
                          n163 = Bundle By Name(cluster=T2 {"identifier"=0, "timestamp"=timestamp(0 s since 1904-01-01), "payload"=[]} ("can cluster"), "identifier"=w229, "payload"=w228, "timestamp"=w232) -> (w235:T2)
                          n164 = global read "rio_Global.vi" "Car_name"() -> (w227:string)
                          n165 = call "can decoder.vi"("can cluster"=w235, "name"=w227) -> ()  [unwired: 10 in]
                        }
                      }
                      frame #1 {
                        n166 = Array Size(array=w259) -> (size(s)=w260:i32[])
                        n167 = global read "rio_Global.vi" "LCM_CAN_RAW_SNAP"() -> (w257:T5)
                        n168 = Multiply Array Elements(1:w260) -> (0:w251:i32)
                        n169 = Get Date/Time In Seconds() -> (seconds since 1Jan1904=w255:timestamp)
                        n170 = To Double Precision Float(number=w255) -> (double precision float=w254:dbl)
                        n171 = Reshape Array(w259, w251) -> (w250:u8[])
                        n172 = Unbundle By Name(w257) -> ("hash"=w252:i64)
                        n173 = Multiply(x=w254, y=1000000.0) -> (x*y=w256:dbl)
                        n174 = call "hash.vi"("input"=w252) -> ("output"=w258:i64)  [unwired: 10 in]
                        n175 = To Quad Integer(1:w256) -> (0:w244:i64)
                        n176 = Bundle(cluster=w257, "hash"=w258, "sys time"=w244, "size"=w251, "data"=w250) -> (w248:T5)
                        n177 = global read "rio_Global.vi" "Car_name"() -> (w245:string)
                        n178 = Flatten To String(anything=w248, prepend array or string size? (T)=FALSE) -> (data string=w246:string)  [unwired: 2 in, 2 out]
                        n179 = global read "rio_Global.vi" "LCM"() -> (w247:T4)
                        n180 = call "LCM_send.vi"("DATA"=w246, "ID"=w245, "LCM"=w247) -> ()  [unwired: 7 in, 2 out]
                      }
                      frame #2 {
                        n181 = global read "rio_Global.vi" "LCM_CAN_T"() -> (w274:T6)
                        n182 = global read "rio_Global.vi" "C_VS_CAN"() -> (w263:dbl)
                        n183 = global read "rio_Global.vi" "C_mdps str_ang"() -> (w272:dbl)
                        n184 = global read "rio_Global.vi" "C_mdps torque"() -> (w265:dbl)
                        n185 = local read "vgain"() -> (w264:dbl)
                        n186 = Unbundle By Name(w274) -> ("hash"=w275:i64)
                        n187 = Multiply(x=w263, y=w264) -> (x*y=w262:dbl)
                        n188 = call "hash.vi"("input"=w275) -> ("output"=w273:i64)  [unwired: 10 in]
                        n189 = global read "rio_Global.vi" "time"() -> (w261:dbl)
                        n190 = Bundle By Name(cluster=w274, "hash"=w273, "mdps str_ang"=w272, "time"=w261, "VS_CAN"=w262, "sys time"=w271, "mdps torque"=w265) -> (w268:T6)
                        n191 = Flatten To String(anything=w268, prepend array or string size? (T)=FALSE) -> (data string=w267:string)  [unwired: 2 in, 2 out]
                        n192 = global read "rio_Global.vi" "LCM"() -> (w270:T4)
                        n193 = call "LCM_send.vi"("DATA"=w267, "ID"="CAN_T", "LCM"=w270) -> ()  [unwired: 7 in, 2 out]
                      }
                    }
                  }
                  frame True {
                  }
                }
              }
            }
          }
        }
      }
    }
  }
  n194 = flat-sequence {
    frame #0 {
      n195 = local write "Manual Steering torque"(0.0 ("Ref_vel_planner")) -> ()
      n196 = local write "Steer input"(FALSE ("Steer input")) -> ()
      n197 = local write "Velocity input"(FALSE ("GPS init")) -> ()
      n198 = local write "Manual Speed"(20.0 ("manual Speed")) -> ()
      n199 = global write "rio_Global.vi" "lane width"(3.5 ("lane width")) -> ()
    }
    frame #1 {
      n200 = while {
        stop <- FALSE stop-if-true
        n201 = flat-sequence {
          tunnel: [w416] -> w293
          tunnel: w293 -> [w468]
          frame #0 {
            n202 = Wait Until Next ms Multiple(millisecond multiple=u32 10) -> (millisecond timer value=w298:u32)
            n203 = feedback #3(w298) -> (w297:u32)
            n204 = feedback-in #3(w298) -> ()
            n205 = Subtract(x=w298, y=w297) -> (x-y=w296:u32)
            n206 = To Long Integer(number=w296) -> (32bit integer=→"Con_time 10":i32)
          }
          frame #1 {
            n207 = disable-structure shown="Enabled" {
              disable-tunnel: [w303 "Mobileye" ("ID")] -> w301
              disable-tunnel: [w302 _] -> w300
              frame Enabled {
                n208 = global read "rio_Global.vi" "LCM PC"() -> (w304:T4)
                n209 = call "LCM_read.vi"("LCM"=w304) -> ("data"=w302:string, "ID"=w303:string)  [unwired: 7 in, 2 out]
              }
              frame Disabled {
              }
            }
            n210 = case shown="\"CON_INPUT_T\"" w301 {
              tunnel: w300 -> [_ w397 _]
              frame "Mobileye" {
                n211 = flat-sequence {
                  frame #0 {
                    w312 = 2 ("index")
                    w315 = 2 ("index")
                    n212 = global read "rio_Global.vi" "M_lane_right"() -> (w307:dbl[])
                    n213 = global read "rio_Global.vi" "M_lane_left"() -> (w308:dbl[])
                    n214 = Index Array(array=w308, index=w315) -> (element=w314:dbl)
                    n215 = Index Array(array=w307, index=w312) -> (element=w313:dbl)
                    n216 = Greater Or Equal?(x=w314, y=w315) -> (x >= y?=w309:bool)
                    n217 = Greater Or Equal?(x=w313, y=w312) -> (x >= y?=w310:bool)
                    n218 = Or(x=w309, y=w310) -> (x .or. y?=w311:bool)
                    n219 = case shown="True" w311 {
                      tunnel: w310 -> [_ w343]
                      tunnel: [w316 w332] -> w306
                      tunnel: w309 -> [_ w346]
                      tunnel: w308 -> [_ w337]
                      tunnel: w307 -> [_ w336]
                      frame False {
                        n220 = global read "rio_Global.vi" "Ref_str_torque"() -> (w317:dbl)
                        n221 = Multiply(x=w317, y=0.997) -> (x*y=w316:dbl)
                      }
                      frame True {
                        n222 = disable-structure shown="Enabled" {
                          disable-tunnel: [w351 w354] -> w342
                          disable-tunnel: [w350 w376] -> w340
                          disable-tunnel: w337 -> [w349 w385]
                          disable-tunnel: w336 -> [w348 w355]
                          frame Disabled {
                            n223 = Index Array(array=w349, index=5) -> (element=w350:dbl)
                            n224 = Index Array(array=w348, index=5) -> (element=w351:dbl)
                          }
                          frame Enabled {
                            n225 = global read "rio_Global.vi" "C_VS_CAN"() -> (w384:dbl)
                            n226 = global read "rio_Global.vi" "C_VS_CAN"() -> (w360:dbl)
                            n227 = In Range and Coerce(upper limit=45.0, x=w384, lower limit=15.0) -> (coerced(x)=w373:dbl)  [unwired: 1 out]
                            n228 = In Range and Coerce(upper limit=45.0, x=w360, lower limit=15.0) -> (coerced(x)=w370:dbl)  [unwired: 1 out]
                            n229 = Index Array(array=w385, index #1=7 ("index"), index #2=6 ("index"), index #3=9 ("index"), index #4=5 ("index")) -> (element #1=w381:dbl, element #2=w374:dbl, element #3=w372:dbl, element #4=w377:dbl)
                            n230 = Index Array(array=w355, index #1=7 ("index"), index #2=6 ("index"), index #3=9 ("index"), index #4=5 ("index")) -> (element #1=w363:dbl, element #2=w369:dbl, element #3=w371:dbl, element #4=w367:dbl)
                            n231 = Square(x=w373) -> (x^2=w375:dbl)
                            n232 = Square(x=w370) -> (x^2=w368:dbl)
                            n233 = Multiply(x=w375, y=w374) -> (x*y=w379:dbl)
                            n234 = Multiply(x=w373, y=w372) -> (x*y=w378:dbl)
                            n235 = Multiply(x=w368, y=w369) -> (x*y=w365:dbl)
                            n236 = Multiply(x=w370, y=w371) -> (x*y=w366:dbl)
                            n237 = Compound Arithmetic op=MULTIPLY(w381, w375, w373) -> (w380:dbl)
                            n238 = Compound Arithmetic op=MULTIPLY(w363, w368, w370) -> (w364:dbl)
                            n239 = Compound Arithmetic op=ADD(w380, w379, w378, w377) -> (w376:dbl)
                            n240 = Compound Arithmetic op=ADD(w364, w365, w366, w367) -> (w354:dbl)
                          }
                        }
                        n241 = global read "rio_Global.vi" "C_VS_CAN"() -> (w335:dbl)
                        n242 = global read "rio_Global.vi" "lane width"() -> (w339:dbl)
                        n243 = Square(x=w335) -> (x^2=w334:dbl)
                        n244 = Add(x=w340, y=w339) -> (x+y=w338:dbl)
                        n245 = Subtract(x=w342, y=w339) -> (x-y=w344:dbl)
                        n246 = Divide(x=w334, y=-28800.0) -> (x/y=w331:dbl)
                        n247 = global read "rio_Global.vi" "C_Right light"() -> (w323:bool)
                        n248 = Select(t=w340, s=w346, f=w344) -> (s? t:f=w345:dbl)
                        n249 = Select(t=w342, s=w343, f=w338) -> (s? t:f=w341:dbl)
                        n250 = global read "rio_Global.vi" "C_Left light"() -> (w321:bool)
                        n251 = Negate(x=w345) -> (-x=w347:dbl)
                        n252 = Multiply(x=w331, y=4.499999999999998 ("invgain>1")) -> (x*y=w330:dbl)
                        n253 = Subtract(x=w347, y=w341) -> (x-y=w320:dbl)
                        n254 = Exclusive Or(1:w323, 2:w321) -> (0:w322:bool)
                        n255 = Exponential(1:w330) -> (0:w327:dbl)
                        n256 = case shown="True" w322 {
                          tunnel: w321 -> [_ w396]
                          tunnel: [w390 w391] -> w319
                          tunnel: w320 -> [w390 w393]
                          frame False {
                          }
                          frame True {
                            n257 = Select(t=1.0, s=w396, f=-1.0) -> (s? t:f=w392:dbl)
                            n258 = Add(x=w393, y=w392) -> (x+y=w391:dbl)
                          }
                        }
                        n259 = Multiply(x=w327, y=0.125) -> (x*y=w326:dbl)
                        n260 = Max & Min(x=w326, y=0.01) -> (max(x,y)=w325:dbl)  [unwired: 1 out]
                        n261 = Multiply(x=w319, y=w325) -> (x*y=w332:dbl)
                      }
                    }
                    n262 = global write "rio_Global.vi" "Ref_str_torque"(w306) -> ()
                  }
                }
              }
              frame "CON_INPUT_T" {
                n263 = global read "rio_Global.vi" "CON_INPUT_T 2"() -> (w399:T8)
                n264 = Unflatten From String(type=w399, binary string=w397, data includes array or string size? (T)=FALSE) -> (value=w398:T8, error out=w400:errorcluster)  [unwired: 2 in, 1 out]
                n265 = case shown="Error" w400 {
                  tunnel: w398 -> [w404 _]
                  tunnel: w397 -> [_ w405]
                  frame No Error {
                    n266 = Unbundle By Name(w404) -> ("ref_vel"=w403:dbl, "ref_steer"=w402:dbl)
                    n267 = global write "rio_Global.vi" "Ref_VS"(w403) -> ()
                    n268 = global write "rio_Global.vi" "Ref_str_ang"(w402) -> ()
                  }
                  frame Error {
                    n269 = global read "rio_Global.vi" "CON_INPUT_T"() -> (w407:T9)
                    n270 = Unflatten From String(type=w407, binary string=w405, data includes array or string size? (T)=FALSE) -> (value=w406:T9, error out=w408:errorcluster)  [unwired: 2 in, 1 out]
                    n271 = case shown="No Error" w408 {
                      tunnel: w406 -> [w412 _]
                      frame No Error {
                        n272 = Unbundle By Name(w412) -> ("ref_vel"=w411:dbl, "ref_steer"=w410:dbl)
                        n273 = global write "rio_Global.vi" "Ref_VS"(w411) -> ()
                        n274 = global write "rio_Global.vi" "Ref_str_ang"(w410) -> ()
                      }
                      frame Error {
                      }
                    }
                  }
                }
              }
              frame Default {
              }
            }
          }
          frame #2 {
            n275 = local read "Con_time 10"() -> (w422:i32)
            n276 = global read "rio_Global.vi" "C_VS_CAN"() -> (w414:dbl)
            n277 = global read "rio_Global.vi" "C_MCP"() -> (→"C_MCP":dbl)
            n278 = global read "rio_Global.vi" "Ref_VS"() -> (w417:dbl)
            n279 = global read "rio_Global.vi" "C_APV"() -> (→"C_APV":dbl)
            n280 = global read "rio_Global.vi" "Car_name"() -> (w418:string)
            n281 = local read "vgain"() -> (w415:dbl)
            n282 = Select(t=w417, s="Velocity input", f="Manual Speed") -> (s? t:f=w427:dbl)
            n283 = To Double Precision Float(number=w422) -> (double precision float=w423:dbl)
            n284 = Multiply(x=w414, y=w415) -> (x*y=→"VS_CAN":dbl)
            n285 = case shown="\"Prius\"" w418 {
              tunnel: w427 -> [w431 w445]
              tunnel: [w430 w446] -> w416
              frame Default {
                n286 = global read "rio_Global.vi" "C_gear selector disp"() -> (w432:u8)
                n287 = case shown="1..3, 5" w432 {
                  tunnel: w431 -> [_ w435 w439]
                  tunnel: [_ w434 w438] -> w430
                  frame 0, Default {
                  }
                  frame 1..3, 5 {
                    n288 = Greater Than 0?(x=w435) -> (x > 0?=w436:bool)
                    n289 = Select(t=w435, s=w436, f=0.0) -> (s? t:f=w434:dbl)
                  }
                  frame 7 {
                    n290 = Less Than 0?(x=w439) -> (x < 0?=w440:bool)
                    n291 = Select(t=w439, s=w440, f=0.0) -> (s? t:f=w438:dbl)
                  }
                }
              }
              frame "Prius" {
                n292 = Sign(1:w445) -> (0:w444:dbl)
                n293 = global read "rio_Global.vi" "C_gear selector disp"() -> (w442:u8)
                n294 = To Long Integer(number=w444) -> (32bit integer=w443:i32)
                n295 = case shown="1" w443 {
                  tunnel: [w448 _ w454] -> w441
                  tunnel: w442 -> [w451 _ w457]
                  frame -1 {
                    n296 = Not Equal?(x=w451, y=u8 1) -> (x != y?=w450:bool)
                    n297 = Select(t=-2.0 ("element"), s=w450, f=0.0) -> (s? t:f=w448:dbl)
                  }
                  frame 0, Default {
                  }
                  frame 1 {
                    n298 = Not Equal?(x=w457, y=u8 3) -> (x != y?=w455:bool)
                    n299 = Select(t=2.0 ("element"), s=w455, f=0.0) -> (s? t:f=w454:dbl)
                  }
                }
                n300 = case shown="3" w442 {
                  tunnel: [_ w459 w464] -> w446
                  tunnel: w445 -> [_ w461 w465]
                  frame 0, Default {
                    # "P,N"
                  }
                  frame 3 {
                    # "D"
                    n301 = Greater Than 0?(x=w461) -> (x > 0?=w462:bool)
                    n302 = Select(t=w461, s=w462, f=0.0) -> (s? t:f=w459:dbl)
                  }
                  frame 1 {
                    # "R"
                    n303 = Less Than 0?(x=w465) -> (x < 0?=w466:bool)
                    n304 = Select(t=w465, s=w466, f=0.0) -> (s? t:f=w464:dbl)
                  }
                }
                n305 = global write "rio_Global.vi" "Shift control"(w441) -> ()
              }
            }
            "Ref_VS" <- w416
            n306 = Multiply(x=w423, y=0.001) -> (x*y=w421:dbl)
            n307 = Max & Min(x=w421, y=0.005) -> (max(x,y)=→"con_dt":dbl)  [unwired: 1 out]
          }
          frame #3 {
            n308 = disable-structure shown="Enabled" {
              disable-tunnel: w468 -> [w481 w522]
              disable-tunnel: [w480 w521] -> w467
              frame Disabled {
                n309 = flat-sequence {
                  tunnel: [w483] -> w480
                  tunnel: w481 -> [w482]
                  frame #0 {
                    n310 = global read "rio_Global.vi" "C_VS_CAN"() -> (w485:dbl)
                    n311 = Subtract(x=w482, y=w485) -> (x-y=w484:dbl)
                    n312 = Less?(x=w484, y=-2.0 ("lower limit")) -> (x < y?=w486:bool)
                    n313 = case shown="True" w486 {
                      tunnel: [w488 w510] -> w483
                      tunnel: w482 -> [w492 w511]
                      tunnel: w484 -> [w494 w502]
                      frame False {
                        n314 = Greater?(x=w494, y=1.0) -> (0:w497:bool)
                        n315 = global read "rio_Global.vi" "PWM Brake"() -> (w501:dbl)
                        n316 = Equal To 0?(x=w492) -> (x = 0?=w491:bool)
                        n317 = Multiply(x=w501, y=0.999) -> (x*y=w499:dbl)
                        n318 = Max & Min(x=w499, y=1000.0) -> (max(x,y)=w495:dbl)  [unwired: 1 out]
                        n319 = Select(t=1000.0, s=w497, f=w495) -> (s? t:f=w489:dbl)
                        n320 = Select(t=2000.0, s=w491, f=w489) -> (s? t:f=w488:dbl)
                      }
                      frame True {
                        w508 = 0.5 ("gain brake")
                        w517 = 10.0 ("y")
                        n321 = Absolute Value(x=w502) -> (abs(x)=w519:dbl)
                        n322 = Add(x=w519, y=w517) -> (x+y=w518:dbl)
                        n323 = Multiply(x=w518, y=w517) -> (x*y=w516:dbl)
                        n324 = Threshold 1D Array(2:w516, 3:dbl[] [10.0, 15.0, 25.0, 50.0, 80.0, 120.0, 170.0, 230.0, 290.0, 350.0, 420.0]) -> (0:w514:dbl)  [unwired: 1 in]
                        n325 = global read "rio_Global.vi" "PWM Brake"() -> (w506:dbl)
                        n326 = Interpolate 1D Array(1:w514, 2:dbl[] [1000.0, 1100.0, 1200.0, 1300.0, 1400.0, 1500.0, 1600.0, 1700.0, 1800.0, 1900.0, 2000.0]) -> (0:w509:dbl)
                        n327 = Decrement(x=w508) -> (x-1=w507:dbl)
                        n328 = Multiply(x=w509, y=w508) -> (x*y=w504:dbl)
                        n329 = Multiply(x=w507, y=w506) -> (x*y=w505:dbl)
                        n330 = Subtract(x=w504, y=w505) -> (x-y=w503:dbl)
                        n331 = Equal To 0?(x=w511) -> (x = 0?=w512:bool)
                        n332 = Select(t=2000.0, s=w512, f=w503) -> (s? t:f=w510:dbl)
                      }
                    }
                  }
                }
              }
              frame Enabled {
                n333 = flat-sequence {
                  tunnel: [w524] -> w521
                  tunnel: w522 -> [w525]
                  frame #0 {
                    n334 = local read "VS_CAN"() -> (w523:dbl)
                    n335 = Subtract(x=w525, y=w523) -> (x-y=w526:dbl)
                    n336 = Less?(x=w526, y=-2.0 ("lower limit")) -> (x < y?=w527:bool)
                    n337 = case shown="True" w527 {
                      tunnel: [w533 w555] -> w524
                      tunnel: w525 -> [w530 w566]
                      tunnel: w526 -> [w541 w558]
                      tunnel: w523 -> [w529 _]
                      frame False {
                        n338 = Equal?(x=1.0, y=w530) -> (x = y?=w538:bool)
                        n339 = Less?(x=w529, y=0.1 ("x")) -> (x < y?=w534:bool)
                        n340 = global read "rio_Global.vi" "PWM Brake"() -> (w550:dbl)
                        n341 = And(x=w538, y=w534) -> (x .and. y?=w537:bool)
                        n342 = Equal To 0?(x=w530) -> (x = 0?=w543:bool)
                        n343 = Multiply(x=w550, y=0.9995 ("brake relase gain")) -> (x*y=w549:dbl)
                        n344 = Greater?(x=w541, y=1.2) -> (0:w547:bool)
                        n345 = Max & Min(x=w549, y=1000.0) -> (max(x,y)=w545:dbl)  [unwired: 1 out]
                        n346 = Select(t=1000.0, s=w547, f=w545) -> (s? t:f=w532:dbl)
                        n347 = Select(t=1200.0, s=w537, f=w532) -> (s? t:f=w531:dbl)
                        n348 = Select(t=1900.0, s=w543, f=w531) -> (s? t:f=w533:dbl)
                      }
                      frame True {
                        w564 = 0.5 ("gain brake")
                        n349 = Absolute Value(x=w558) -> (abs(x)=w557:dbl)
                        n350 = Threshold 1D Array(2:w557, 3:dbl[] [0.1, 0.5, 1.0, 1.5, 2.0, 3.0, 4.0, 5.0, 6.0, 7.0, 8.0, 9.0] ("Array 2")) -> (0:w569:dbl)  [unwired: 1 in]
                        n351 = global read "rio_Global.vi" "PWM Brake"() -> (w562:dbl)
                        n352 = Interpolate 1D Array(1:w569, 2:dbl[] [1330.0, 1340.0, 1350.0, 1370.0, 1380.0, 1400.0, 1450.0, 1500.0, 1550.0, 1700.0, 1750.0, 1900.0] ("Array")) -> (0:w565:dbl)
                        n353 = Decrement(x=w564) -> (x-1=w563:dbl)
                        n354 = Multiply(x=w565, y=w564) -> (x*y=w560:dbl)
                        n355 = Multiply(x=w563, y=w562) -> (x*y=w561:dbl)
                        n356 = Subtract(x=w560, y=w561) -> (x-y=w556:dbl)
                        n357 = Equal To 0?(x=w566) -> (x = 0?=w567:bool)
                        n358 = disable-structure shown="Enabled" {
                          disable-tunnel: [w571 w572] -> w553
                          disable-tunnel: w556 -> [w571 w585]
                          disable-tunnel: w557 -> [_ w577]
                          frame Disabled {
                          }
                          frame Enabled {
                            n359 = Multiply(x=w577, y=120.0 ("brake p gain")) -> (x*y=w583:dbl)
                            n360 = local read "con_dt"() -> (w580:dbl)
                            n361 = Add(x=w585, y=w583) -> (x+y=w574:dbl)
                            n362 = Multiply(x=w580, y=4.0) -> (x*y=w579:dbl)
                            n363 = call <vilib>:"Derivative x(t) PtByPt.vi"("initialize"=FALSE, "dt"=w579, "initial condition"=0.0, "x"=w577) -> ("dx/dt"=w575:dbl)  [unwired: 1 out]
                            n364 = Multiply(x=30.0 ("bake d gain"), y=w575) -> (x*y=w573:dbl)
                            n365 = Add(x=w574, y=w573) -> (x+y=w572:dbl)
                          }
                        }
                        n366 = In Range and Coerce(upper limit=1900.0, x=w553, lower limit=1000.0) -> (coerced(x)=w551:dbl)  [unwired: 1 out]
                        n367 = Select(t=1900.0, s=w567, f=w551) -> (s? t:f=w555:dbl)
                      }
                    }
                  }
                }
              }
            }
            n368 = global read "rio_Global.vi" "Car_name"() -> (w469:string)
            n369 = Not Equal To 0?(x=w468) -> (x != 0?=w470:bool)
            n370 = case shown="\"Prius111\"" w469 {
              tunnel: [w607 w626 w654] -> w474
              tunnel: w468 -> [w606 w625 w653]
              frame "Santafe" {
                w590 = 5.0 ("gain accel")
                w598 = 12.0 ("y")
                n371 = Subtract(x=w606, y=20.0) -> (x-y=w602:dbl)
                n372 = global read "rio_Global.vi" "C_VS_CAN"() -> (w587:dbl)
                n373 = Multiply(x=w602, y=0.4) -> (x*y=w600:dbl)
                n374 = Subtract(x=w606, y=w587) -> (x-y=w586:dbl)
                n375 = Add(x=w600, y=w598) -> (x+y=w599:dbl)
                n376 = In Range and Coerce(upper limit=35.0, x=w599, lower limit=w598) -> (coerced(x)=w596:dbl)  [unwired: 1 out]
                n377 = In Range and Coerce(upper limit=20.0, x=w586, lower limit=-10.0) -> (coerced(x)=w595:dbl)  [unwired: 1 out]
                n378 = Multiply(x=w595, y=w596) -> (x*y=w588:dbl)
                n379 = Multiply(x=w588, y=w590) -> (x*y=w592:dbl)
                n380 = Decrement(x=w590) -> (x-1=w589:dbl)
                n381 = feedback #4(0.0) -> (w593:dbl)
                n382 = feedback-in #4(w588) -> ()
                n383 = Multiply(x=w589, y=w593) -> (x*y=w591:dbl)
                n384 = Subtract(x=w592, y=w591) -> (x-y=w607:dbl)
              }
              frame "Prius111" {
                w617 = 0.09999999999999998 ("lpf gain speed")
                n385 = global read "rio_Global.vi" "C_VS_CAN"() -> (w610:dbl)
                n386 = feedback #5(w610) -> (w611:dbl)
                n387 = feedback-in #5(w610) -> ()
                n388 = Subtract(x=w610, y=w611) -> (x-y=w621:dbl)
                n389 = Multiply(x=w621, y=5.0) -> (x*y=w620:dbl)
                n390 = Add(x=w610, y=w620) -> (x+y=w619:dbl)
                n391 = Subtract(x=w625, y=w619) -> (x-y=w624:dbl)
                n392 = Decrement(x=w617) -> (x-1=w616:dbl)
                n393 = Multiply(x=45.0 ("x 2"), y=w624) -> (x*y=w618:dbl)
                n394 = Multiply(x=w618, y=w617) -> (x*y=w615:dbl)
                n395 = feedback #6(0.0) -> (w613:dbl)
                n396 = Multiply(x=w616, y=w613) -> (x*y=w614:dbl)
                n397 = Subtract(x=w615, y=w614) -> (x-y=w609:dbl)
                n398 = feedback-in #6(w609) -> ()
                n399 = Multiply(x=0.1, y=w609) -> (x*y=w626:dbl)
              }
              frame "Avante", Default {
                n400 = local read "VS_CAN"() -> (w627:dbl)
                n401 = Subtract(x=w653, y=w627) -> (x-y=w652:dbl)
                n402 = In Range and Coerce(upper limit=20.0, x=w652, lower limit=-999.0) -> (coerced(x)=w632:dbl)  [unwired: 1 out]
                n403 = local read "con_dt"() -> (w630:dbl)
                n404 = feedback #7(w632) -> (w634:dbl)
                n405 = feedback-in #7(w632) -> ()
                n406 = Absolute Value(x=w632) -> (abs(x)=w639:dbl)
                n407 = feedback #8(0.0) -> (w648:dbl)
                n408 = Multiply(x=w648, y=0.98) -> (x*y=w642:dbl)
                n409 = Multiply(x=w632, y=0.01) -> (x*y=w649:dbl)
                n410 = Subtract(x=w632, y=w634) -> (x-y=w633:dbl)
                n411 = Add(x=w642, y=w649) -> (x+y=w643:dbl)
                n412 = feedback-in #8(w643) -> ()
                n413 = Greater?(x=w639, y=1.0) -> (0:w636:bool)
                n414 = Multiply(x=w630, y=4.0) -> (x*y=w628:dbl)
                n415 = Divide(x=w633, y=w628) -> (x/y=w631:dbl)
                n416 = Select(t=w632, s=w636, f=0.0) -> (s? t:f=w646:dbl)
                n417 = Build Array(w646, w643, w631) -> (w645:dbl[])
                n418 = Multiply(x="V_PID_gain", y=w645) -> (x*y=w644:dbl[])
                n419 = Add Array Elements(numeric array=w644) -> (sum=w654:dbl)
              }
            }
            n420 = global read "rio_Global.vi" "C_Brake"() -> (w472:bool)
            n421 = local read "T out"() -> (w476:i32)
            n422 = local read "T init"() -> (w477:i32)
            n423 = Greater Or Equal?(x=w477, y=w476) -> (x >= y?=w473:bool)
            n424 = Not(x=w472) -> (.not. x?=w471:bool)
            n425 = Compound Arithmetic op=AND(w473, w471, w470) -> (w475:bool)
            n426 = case shown="True" w475 {
              tunnel: [1000.0 ("Numeric") w670] -> w478
              tunnel: w474 -> [_ w672]
              tunnel: w476 -> [w656 _]
              tunnel: [_ TRUE] -> w479
              frame False {
                n427 = local read "T init"() -> (w657:i32)
                n428 = Less Or Equal?(x=w657, y=w656) -> (x <= y?=w658:bool)
                n429 = case shown="False" w658 {
                  tunnel: w656 -> [_ w661]
                  frame False {
                    n430 = local write "T init"(1 ("T init")) -> ()
                  }
                  frame True {
                    n431 = local read "T init"() -> (w664:i32)
                    n432 = Increment(x=w664) -> (x+1=w663:i32)
                    n433 = Max & Min(x=w663, y=w661) -> (min(x,y)=w662:i32)  [unwired: 1 out]
                    n434 = local write "T init"(w662) -> ()
                  }
                }
              }
              frame True {
                n435 = To Long Integer(number=w672) -> (32bit integer=w674:i32)
                n436 = Multiply(x=10.0, y=w672) -> (x*y=w669:dbl)
                n437 = Add(x=w674, y=20) -> (x+y=w676:i32)
                "T out" <- w676
                n438 = Add(x=w669, y=1000.0 ("PWM GAS")) -> (x+y=w667:dbl)
                n439 = Increment(x=w676) -> (x+1=→"T init":i32)
                n440 = In Range and Coerce(upper limit=1600.0, x=w667, lower limit=1000.0 ("x")) -> (coerced(x)=w670:dbl)  [unwired: 1 out]
              }
            }
            n441 = global write "rio_Global.vi" "Solenoid"(w479) -> ()
            n442 = global write "rio_Global.vi" "PWM GAS"(w478) -> ()
            n443 = disable-structure shown="Enabled" {
              disable-tunnel: w467 -> [w655 _]
              frame Enabled {
                n444 = global write "rio_Global.vi" "PWM Brake"(w655) -> ()
              }
              frame Disabled {
              }
            }
          }
          frame #4 {
            n445 = disable-structure shown="Disabled" {
              disable-tunnel: [w781 "Dial"] -> w679
              frame Enabled {
                n446 = global read "rio_Global.vi" "Ref_str_ang"() -> (w781:dbl)
              }
              frame Disabled {
              }
            }
            n447 = disable-structure shown="Enabled" {
              disable-tunnel: [_ w738] -> w678
              disable-tunnel: w679 -> [_ w723]
              frame Disabled {
                w708 = 0.6000000000000001 ("y")
                n448 = Absolute Value() -> (x=w683:dbl, abs(x)=w702:dbl)
                n449 = Not A Number/Path/Refnum?(number/path/refnum=w683) -> (NaN/Path/Refnum?=w711:bool)
                n450 = Select(t=0.0, s=w711, f=w683) -> (s? t:f=w710:dbl)
                n451 = Multiply(x=w702, y=-0.02) -> (x*y=w700:dbl)
                n452 = Add(x=w700, y=1.1) -> (x+y=w698:dbl)
                n453 = global read "rio_Global.vi" "C_mdps str_ang"() -> (w687:dbl)
                n454 = In Range and Coerce(upper limit=0.22, x=w698, lower limit=0.08) -> (coerced(x)=w695:dbl)  [unwired: 1 out]
                n455 = Negate(x=w695) -> (-x=w693:dbl)
                n456 = Bundle By Name(cluster=T7 {"proportional gain (Kc)"=-0.1, "integral time (Ti, min)"=0.0, "derivative time (Td, min)"=0.0} ("PID gains"), "proportional gain (Kc)"=w693) -> (w692:T7)
                n457 = Not A Number/Path/Refnum?(number/path/refnum=w687) -> (NaN/Path/Refnum?=w715:bool)
                n458 = Select(t=0.0, s=w715, f=w687) -> (s? t:f=w713:dbl)
                n459 = call-poly <vilib>:"PID.vi"("output range"=cluster{"output high":dbl, "output low":dbl} {"output high"=5.0, "output low"=-5.0}, "dt (s)"=-1.0, "PID gains"=w692, "process variable"=w713, "setpoint"=w710) -> ("output"=w709:dbl)  [unwired: 5 in, 1 out]
                n460 = Decrement(x=w708) -> (x-1=w707:dbl)
                n461 = Multiply(x=w709, y=w708) -> (x*y=w704:dbl)
                n462 = global read "rio_Global.vi" "C_mdps torque"() -> (w685:dbl)
                n463 = feedback #9(0.0) -> (w706:dbl)
                n464 = Multiply(x=w707, y=w706) -> (x*y=w705:dbl)
                n465 = Subtract(x=w704, y=w705) -> (x-y=w689:dbl)
                n466 = Not A Number/Path/Refnum?(number/path/refnum=w689) -> (NaN/Path/Refnum?=w691:bool)
                n467 = Select(t=0.0, s=w691, f=w689) -> (s? t:f=w688:dbl)
                n468 = feedback-in #9(w688) -> ()
                n469 = Multiply(x=-0.05 ("x 5"), y=w685) -> (x*y=w684:dbl)
                n470 = Multiply(x=0.1 ("x 2"), y=w688) -> (x*y=w716:dbl)
                n471 = Add(x=w716, y=w684) -> ()  [unwired: 1 out]
              }
              frame Enabled {
                n472 = global read "rio_Global.vi" "C_mdps str_ang"() -> (w733:dbl)
                n473 = disable-structure shown="Enabled" {
                  disable-tunnel: [w770 w771] -> w722
                  disable-tunnel: w733 -> [w769 w771]
                  frame Enabled {
                    w763 = 0.8 ("lpf gain 2")
                    n474 = Multiply(x=w769, y=w763) -> (x*y=w767:dbl)
                    n475 = Decrement(x=w763) -> (x-1=w768:dbl)
                    n476 = feedback #10(0.0) -> (w765:dbl)
                    n477 = Multiply(x=w768, y=w765) -> (x*y=w766:dbl)
                    n478 = Subtract(x=w767, y=w766) -> (x-y=w770:dbl)
                    n479 = feedback-in #10(w770) -> ()
                  }
                  frame Disabled {
                  }
                }
                n480 = local read "con_dt"() -> (w736:dbl)
                n481 = Multiply(x=w736, y=4.0) -> (x*y=w735:dbl)
                n482 = Add(x=w723, y=w722) -> (x+y=w737:dbl)
                n483 = disable-structure shown="Enabled" {
                  disable-tunnel: w737 -> [w755 w760]
                  disable-tunnel: [w754 w760] -> w726
                  frame Enabled {
                    n484 = Absolute Value(x=w755) -> (abs(x)=w759:dbl)
                    n485 = Greater?(x=w759, y=0.4) -> (0:w757:bool)
                    n486 = Select(t=w755, s=w757, f=0.0) -> (s? t:f=w754:dbl)
                  }
                  frame Disabled {
                  }
                }
                n487 = call <vilib>:"Derivative x(t) PtByPt.vi"("initialize"=FALSE, "dt"=w735, "initial condition"=0.0, "x"=w722) -> ("dx/dt"=w724:dbl)  [unwired: 1 out]
                n488 = local read "con_dt"() -> (w743:dbl)
                n489 = global read "rio_Global.vi" "Car_name"() -> (w721:string)
                n490 = case shown="\"Prius\"" w721 {
                  tunnel: [dbl[] [0.035, 7.5, 0.003] ("STEERING PID_gain_Prius") dbl[] [0.02, 6.5, 0.003] ("STEERING PID_gain_Hyundai")] -> w720
                  frame "Prius" {
                  }
                  frame Default {
                  }
                }
                n491 = Index Array(array=w720, index=0) -> (element=w727:dbl)
                n492 = Reciprocal(x=w727) -> (1/x=w739:dbl)
                n493 = feedback #11(0.0) -> (w742:dbl)
                n494 = Add(x=w726, y=w742) -> (x+y=w744:dbl)
                n495 = call <vilib>:"Integral x(t) PtByPt.vi"("initialize"=FALSE, "dt"=w743, "initial condition"=0.0, "x"=w744) -> ("integral x(t)"=w751:dbl)  [unwired: 1 out]
                n496 = Compound Arithmetic op=MULTIPLY(w751, 0.01 ("x")) -> (w732:dbl)
                n497 = Build Array(w726, w732, w724) -> (w731:dbl[])
                n498 = Multiply(x=w731, y=w720) -> (x*y=w730:dbl[])
                n499 = Add Array Elements(numeric array=w730) -> (sum=w729:dbl)
                n500 = In Range and Coerce(upper limit=0.55, x=w729, lower limit=-0.55) -> (coerced(x)=w741:dbl)  [unwired: 1 out]
                n501 = disable-structure shown="Enabled" {
                  disable-tunnel: w741 -> [w779 w780]
                  disable-tunnel: [w778 w780] -> w738
                  frame Enabled {
                    w772 = 0.8 ("lpf gain")
                    n502 = Multiply(x=w779, y=w772) -> (x*y=w776:dbl)
                    n503 = Decrement(x=w772) -> (x-1=w777:dbl)
                    n504 = feedback #12(0.0) -> (w774:dbl)
                    n505 = Multiply(x=w777, y=w774) -> (x*y=w775:dbl)
                    n506 = Subtract(x=w776, y=w775) -> (x-y=w778:dbl)
                    n507 = feedback-in #12(w778) -> ()
                  }
                  frame Disabled {
                  }
                }
                n508 = Subtract(x=w741, y=w729) -> (x-y=w740:dbl)
                n509 = Multiply(x=w740, y=w739) -> (x*y=w745:dbl)
                n510 = feedback-in #11(w745) -> ()
              }
            }
            n511 = Select(t=w678, s="Steer input", f="Manual Steering torque") -> (s? t:f=w680:dbl)
            n512 = global write "rio_Global.vi" "steering torque"(w680) -> ()
          }
          frame #5 {
            n513 = Get Date/Time In Seconds() -> (seconds since 1Jan1904=w798:timestamp)
            n514 = global read "rio_Global.vi" "LCM_CON_T 2"() -> (w807:T10)
            n515 = To Double Precision Float(number=w798) -> (double precision float=w797:dbl)
            n516 = Unbundle By Name(w807) -> ("hash"=w808:i64)
            n517 = Multiply(x=w797, y=1000000.0) -> (x*y=w801:dbl)
            n518 = global read "rio_Global.vi" "PWM Brake"() -> (w784:dbl)
            n519 = global read "rio_Global.vi" "Ref_str_ang"() -> (w787:dbl)
            n520 = global read "rio_Global.vi" "PWM GAS"() -> (w783:dbl)
            n521 = global read "rio_Global.vi" "Solenoid"() -> (w791:bool)
            n522 = String To IP(1:"192.168.100.200") -> (0:w792:u32)
            n523 = To Quad Integer(1:w801) -> (0:w799:i64)
            n524 = call "hash.vi"("input"=w808) -> ("output"=w806:i64)  [unwired: 10 in]
            n525 = local read "Ref_VS"() -> (w788:dbl)
            n526 = global read "rio_Global.vi" "Auto"() -> (w794:bool)
            n527 = global read "rio_Global.vi" "Run"() -> (w793:bool)
            n528 = Bundle By Name(cluster=w807, "hash"=w806, "sys time"=w799, "Auto"=w794, "Run"=w793, "Solenoid"=w791, "T lim"=FALSE, "brk_enc"=u8 0, "B PWM"=w784, "T PWM"=w783, "ref_vel"=w788, "ref_bkr_enc"=0.0, "ref_apv"=0.0, "ref_steer"=w787, "net address"=w792) -> (w796:T10)
            n529 = Flatten To String(anything=w796, prepend array or string size? (T)=FALSE) -> (data string=w803:string)  [unwired: 2 in, 2 out]
            n530 = global read "rio_Global.vi" "LCM"() -> (w805:T4)
            n531 = call "LCM_send.vi"("DATA"=w803, "ID"="CON_T", "LCM"=w805) -> ()  [unwired: 7 in, 2 out]
          }
        }
      }
    }
  }
  n532 = disable-structure shown="Disabled" {
    frame Disabled {
      n533 = flat-sequence {
        frame #0 {
          n534 = for {
            N: 257 -> [_]
            tunnel: [w815] -> w813 mode=indexing
            i -> [w815]
          }
          n535 = Multiply(x=w813, y=0.5) -> (x*y=w811:dbl[])
          "x_view" <- w811
          n536 = Array Subset(array=w811, index=30) -> (w809:dbl[])  [unwired: 1 in]
          n537 = global write "rio_Global.vi" "x_view"(w809) -> ()
        }
        frame #1 {
          n538 = while {
            stop <- FALSE stop-if-true
            n539 = flat-sequence {
              frame #0 {
                n540 = Wait Until Next ms Multiple(millisecond multiple=u32 33) -> ()  [unwired: 1 out]
              }
              frame #1 {
                n541 = local read "x_view"() -> (w818:dbl[])
                n542 = call "mobileye_disp.vi"("x_view"=w818) -> ("XY Graph"=→"XY Graph":cluster{"Y":dbl[], "Y":dbl[]}[])  [unwired: 10 in]
              }
            }
          }
        }
      }
    }
    frame Enabled {
    }
  }
  n543 = flat-sequence {
    tunnel: [w828] -> w1
    tunnel: w1 -> [w841]
    frame #0 {
      w834 = FALSE ("get heading")
      w835 = u64 1
      w832 = 0.0 ("dh_hat")
      n544 = disable-structure shown="Disabled" {
        disable-tunnel: [-29.545 _] -> w826
        frame Disabled {
        }
        frame Enabled {
        }
      }
      n545 = local write "GPS on"(TRUE ("GPS on")) -> ()
      n546 = local write "GPS init"(w834) -> ()
      n547 = call "getecefdcmref.vi"("map name"=T11."KAIST") -> ("XYZ"=w830:dbl[])  [unwired: 10 in, 4 out]
      n548 = local write "ecef ref"(w830) -> ()
      n549 = Multiply(x=3.141592653589793, y=w826) -> (x*y=w824:dbl)
      n550 = Divide(x=w824, y=180.0) -> (x/y=w822:dbl)
      n551 = Replace Array Subset(array=dbl[] [0.0, 0.0, 0.0, 0.0, 0.0] ("pos(i)"), new element=w822, index=3) -> (w828:dbl[])
      "vgain" <- 1.0 ("initH")
      "vcount" <- w835
      "hbias" <- w832
      "hcount" <- w835
      "get heading" <- w834
      "get position" <- w834
      "heading error" <- w832
      "h_gps" <- w832
      "pos error" <- w832
      "POS init" <- TRUE ("POS init")
      "conutpos" <- 0
    }
    frame #1 {
      (unwired) FALSE
      n552 = flat-sequence {
        frame #0 {
          n553 = while {
            shift-right: [w1321] -> w1316
            shift-left: refnum<visa-resource-name> "USB0::0x1546::0x01A8::NI-VISA-1003::1::RAW" ("VISA resource name") -> [w1322]
            stop <- w1320 continue-if-true
            n554 = VISA Open(VISA resource name=w1322) -> (VISA resource name=w1321:refnum<visa-resource-name>, error out=w1320:errorcluster)  [unwired: 4 in]
          }
          n555 = VISA Clear(VISA resource name=w1316) -> (VISA resource name out=w1318:refnum<visa-resource-name>)  [unwired: 1 in, 1 out]
          n556 = property class="Instr"(reference=w1318, "General Settings:Timeout Value"=u32 10) -> (reference out=→"gps1":refnum<visa-resource-name>)  [unwired: 1 in, 1 out]
        }
        frame #1 {
          n557 = while {
            stop <- FALSE stop-if-true
            n558 = local read "gps1"() -> (w1325:refnum<visa-resource-name>)
            n559 = VISA Read(VISA resource name=w1325, byte count=u32 100) -> (read buffer=w1323:string)  [unwired: 1 in, 3 out]
            n560 = case shown="Default" w1323 {
              selector: w1323 -> [_ w1328]
              frame "" {
                n561 = Wait (ms)(milliseconds to wait=u32 20) -> ()  [unwired: 1 out]
              }
              frame Default {
                n562 = local read "ecef ref"() -> (w1329:dbl[])
                n563 = call "nmea.vi"("ecef ref"=w1329, "NMEA"=w1328) -> ("output"=w1331:dbl[], "type"=w1330:u32)  [unwired: 8 in]
                n564 = case shown="1" w1330 {
                  tunnel: w1331 -> [_ w1333 w1393]
                  frame 0, Default {
                  }
                  frame 1 {
                    n565 = global write "rio_Global.vi" "gps_pos 1"(w1333) -> ()
                    n566 = Index Array(array=w1333, index=1) -> (element=w1335:dbl)
                    n567 = Not Equal To 0?(x=w1335) -> (x != 0?=w1332:bool)
                    n568 = case shown="True" w1332 {
                      tunnel: w1333 -> [_ w1337]
                      frame False {
                      }
                      frame True {
                        n569 = First Call?() -> (First Call?: T/F=w1336:bool)
                        n570 = case shown="False" w1336 {
                          tunnel: w1337 -> [w1357 w1370]
                          frame False {
                            n571 = Get Date/Time In Seconds() -> (seconds since 1Jan1904=w1342:timestamp)
                            n572 = To Double Precision Float(number=w1342) -> (double precision float=w1341:dbl)
                            n573 = global read "rio_Global.vi" "LCM_GGA_T"() -> (w1366:T15)
                            n574 = Array To Cluster(array=w1357) -> (cluster=w1365:T16)
                            n575 = Unbundle By Name(w1366) -> ("hash"=w1362:i64)
                            n576 = Multiply(x=w1341, y=1000000.0) -> (x*y=w1339:dbl)
                            n577 = Unbundle(w1365) -> ("output[0]"=w1367:dbl, "output[2]"=w1356:dbl, "output[3]"=w1355:dbl, "output[4]"=w1354:dbl, "output[6]"=w1353:dbl, "output[7]"=w1351:dbl, "output[8]"=w1349:dbl, "output[9]"=w1347:dbl, "output[12]"=w1346:dbl, "output[13]"=w1345:dbl, "output[14]"=w1344:dbl)  [unwired: 4 out]
                            n578 = local read "map name"() -> (w1343:T1)
                            n579 = To Quad Integer(1:w1339) -> (0:w1338:i64)
                            n580 = To Long Integer(number=w1353) -> (32bit integer=w1352:i32)
                            n581 = To Long Integer(number=w1351) -> (32bit integer=w1350:i32)
                            n582 = To Long Integer(number=w1349) -> (32bit integer=w1348:i32)
                            n583 = call "hash.vi"("input"=w1362) -> ("output"=w1361:i64)  [unwired: 10 in]
                            n584 = Bundle(cluster=w1366, "hash"=w1361, "sys time"=w1338, "time"=w1367, "x"=w1356, "y"=w1355, "h"=w1354, "numSV"=w1352, "postype"=w1350, "lag"=w1348, "hordev"=w1347, "lat"=w1346, "lon"=w1345, "hgt"=w1344, "map_idx"=w1343) -> (w1363:T15)
                            n585 = Flatten To String(anything=w1363, prepend array or string size? (T)=FALSE) -> (data string=w1359:string)  [unwired: 2 in, 2 out]
                            n586 = global read "rio_Global.vi" "LCM"() -> (w1358:T4)
                            n587 = call "LCM_send.vi"("DATA"=w1359, "ID"="GGA_1", "LCM"=w1358) -> ()  [unwired: 7 in, 2 out]
                          }
                          frame True {
                            n588 = Index Array(array=w1370, index #1=12 ("index")) -> (element #1=w1375:dbl, element #2=w1379:dbl)  [unwired: 1 in]
                            n589 = for {
                              N: 14 -> [_]
                              tunnel: [w1391] -> w1381 mode=indexing
                              tunnel: [w1390] -> w1383 mode=indexing
                              i -> [w1392]
                              n590 = call "getecefdcmref.vi"("map name"=w1392) -> ("lat"=w1391:dbl, "lon"=w1390:dbl)  [unwired: 10 in, 3 out]
                            }
                            n591 = Multiply(x=w1375, y=3.141592653589793) -> (x*y=w1373:dbl)
                            n592 = Multiply(x=w1379, y=3.141592653589793) -> (x*y=w1377:dbl)
                            n593 = Divide(x=w1373, y=180.0) -> (x/y=w1382:dbl)
                            n594 = Divide(x=w1377, y=180.0) -> (x/y=w1384:dbl)
                            n595 = Subtract(x=w1381, y=w1382) -> (x-y=w1385:dbl[])
                            n596 = Subtract(x=w1383, y=w1384) -> (x-y=w1386:dbl[])
                            n597 = Square(x=w1385) -> (x^2=w1387:dbl[])
                            n598 = Square(x=w1386) -> (x^2=w1388:dbl[])
                            n599 = Add(x=w1387, y=w1388) -> (x+y=w1389:dbl[])
                            n600 = Array Max & Min(array=w1389) -> (min index (indices)=w1368:i32)  [unwired: 3 out]
                            "map name" <- w1368
                            n601 = call "getecefdcmref.vi"("map name"=w1368) -> ("XYZ"=→"ecef ref":dbl[])  [unwired: 10 in, 4 out]
                          }
                        }
                      }
                    }
                  }
                  frame 2 {
                    n602 = flat-sequence {
                      tunnel: w1393 -> [w1395]
                      frame #0 {
                        n603 = Index Array(array=w1395, index=1) -> (element=w1397:dbl)
                        n604 = Not Equal To 0?(x=w1397) -> (x != 0?=w1394:bool)
                        n605 = case shown="True" w1394 {
                          tunnel: w1395 -> [_ w1416]
                          frame False {
                          }
                          frame True {
                            n606 = Get Date/Time In Seconds() -> (seconds since 1Jan1904=w1402:timestamp)
                            n607 = To Double Precision Float(number=w1402) -> (double precision float=w1401:dbl)
                            n608 = global read "rio_Global.vi" "LCM_RMC_T"() -> (w1417:T17)
                            n609 = Unbundle By Name(w1417) -> ("hash"=w1413:i64)
                            n610 = Multiply(x=w1401, y=1000000.0) -> (x*y=w1399:dbl)
                            n611 = Array To Cluster(array=w1416) -> (cluster=w1415:T18)
                            n612 = To Quad Integer(1:w1399) -> (0:w1398:i64)
                            n613 = call "hash.vi"("input"=w1413) -> ("output"=w1412:i64)  [unwired: 10 in]
                            n614 = Unbundle(w1415) -> ("output[0]"=w1407:dbl, "output[2]"=w1406:dbl, "output[4]"=w1405:dbl, "output[5]"=w1404:dbl, "output[6]"=w1403:dbl)  [unwired: 2 out]
                            n615 = Bundle(cluster=w1417, "hash"=w1412, "sys time"=w1398, "time"=w1407, "speed"=w1406, "heading"=w1405, "lat"=w1404, "lon"=w1403) -> (w1408:T17)
                            n616 = Flatten To String(anything=w1408, prepend array or string size? (T)=FALSE) -> (data string=w1410:string)  [unwired: 2 in, 2 out]
                            n617 = global read "rio_Global.vi" "LCM"() -> (w1409:T4)
                            n618 = call "LCM_send.vi"("DATA"=w1410, "ID"="RMC_1", "LCM"=w1409) -> ()  [unwired: 7 in, 2 out]
                          }
                        }
                      }
                    }
                    n619 = global write "rio_Global.vi" "gps_vel 1"(w1393) -> ()
                  }
                }
              }
            }
          }
        }
      }
      n620 = node-c288(i64 10 ("Period")) -> (w840:T12)  [unwired: 3 in]
      n621 = timed-loop {
        shift-right: [w842] -> _
        shift-left: w841 -> [w843]
        timing: w840 -> [_]
        timing-out: [_] -> w839
        stop <- FALSE stop-if-true
        n622 = node-c288() -> ()  [unwired: 1 in]
        n623 = flat-sequence {
          tunnel: [w884] -> w846
          tunnel: w843 -> [w884]
          tunnel: w846 -> [w887]
          tunnel: [w886] -> w845
          tunnel: [w886] -> w844
          tunnel: [w1284] -> w842
          tunnel: w845 -> [w1285]
          tunnel: w844 -> [w1284]
          frame #0 {
            n624 = global read "rio_Global.vi" "time"() -> (w877:dbl)
            n625 = call "Tick Count"() -> ("Tick Count(uSec)"=w882:u32)
            n626 = global read "rio_Global.vi" "C_yaw_rate"() -> (w875:dbl)
            n627 = global read "rio_Global.vi" "C_VS_CAN"() -> (w865:dbl)
            n628 = global read "rio_Global.vi" "time V"() -> (w868:dbl)
            n629 = feedback #13(w877) -> (w878:dbl)
            n630 = feedback-in #13(w877) -> ()
            n631 = feedback #14(w882) -> (w883:u32)
            n632 = feedback-in #14(w882) -> ()
            n633 = Subtract(x=w882, y=w883) -> (x-y=w881:u32)
            n634 = Subtract(x=w877, y=w878) -> (x-y=w852:dbl)
            n635 = feedback #15(w875) -> (w876:dbl)
            n636 = feedback-in #15(w875) -> ()
            n637 = feedback #16(w865) -> (w863:dbl)
            n638 = feedback-in #16(w865) -> ()
            n639 = feedback #17(w868) -> (w869:dbl)
            n640 = feedback-in #17(w868) -> ()
            n641 = Add(x=w875, y=w876) -> (x+y=w874:dbl)
            n642 = Add(x=w865, y=w863) -> (x+y=w866:dbl)
            n643 = Subtract(x=w868, y=w869) -> (x-y=w859:dbl)
            n644 = To Double Precision Float(number=w881) -> (double precision float=w880:dbl)
            n645 = In Range and Coerce(upper limit=0.5, x=w852, lower limit=1e-06) -> (In Range?=w855:bool)  [unwired: 1 out]
            n646 = Multiply(x=w874, y=0.5) -> (x*y=w872:dbl)
            n647 = Multiply(x=w866, y=0.5) -> (x*y=→"vel_ave":dbl)
            n648 = Multiply(x=w880, y=1e-06) -> (x*y=→"dt":dbl)
            n649 = In Range and Coerce(upper limit=0.5, x=w859, lower limit=1e-06) -> (In Range?=w860:bool)  [unwired: 1 out]
            n650 = Multiply(x=w872, y=1.0 ("y 2")) -> (x*y=→"C_yaw_rate":dbl)
            n651 = Select(t=w852, s=w855, f=0.0) -> (s? t:f=→"dt yaw":dbl)
            n652 = Select(t=w859, s=w860, f=0.0) -> (s? t:f=→"dt vel":dbl)
          }
          frame #1 {
            n653 = flat-sequence {
              tunnel: w887 -> [w891]
              tunnel: [w891] -> w885
              tunnel: [w891] -> _
              tunnel: [w1046] -> w886
              tunnel: w885 -> [w1047]
              frame #0 {
                n654 = disable-structure shown="Enabled" {
                  disable-tunnel: [w999 w1030] -> w898
                  disable-tunnel: [w998 w1011] -> w894
                  disable-tunnel: [w970 w1022] -> w897
                  disable-tunnel: [w958 w1018] -> w890
                  disable-tunnel: [_ w1006] -> w888
                  frame Disabled {
                    n655 = global read "rio_Global.vi" "gps_vel 1"() -> (w997:dbl[])
                    n656 = global read "rio_Global.vi" "gps_vel 2"() -> (w976:dbl[])
                    n657 = Index Array(array=w997, index #1=0 ("index"), index #2=1 ("index"), index #3=4 ("index"), index #4=2 ("index")) -> (element #1=w988:dbl, element #2=w993:dbl, element #3=w990:dbl, element #4=w962:dbl)
                    n658 = Index Array(array=w976, index #1=0 ("index"), index #2=1 ("index"), index #3=4 ("index"), index #4=2 ("index")) -> (element #1=w985:dbl, element #2=w980:dbl, element #3=w983:dbl, element #4=w961:dbl)
                    n659 = global read "rio_Global.vi" "C_VS_CAN"() -> (w955:dbl)
                    n660 = global read "rio_Global.vi" "C_VS_CAN"() -> (w1002:dbl)
                    n661 = Add(x=w962, y=w961) -> (x+y=w960:dbl)
                    n662 = Not Equal To 0?(x=w980) -> (x != 0?=w981:bool)
                    n663 = call "angleconv.vi"("deg"=w990) -> ("rad"=w973:dbl)  [unwired: 9 in, 1 out]
                    n664 = call "angleconv.vi"("deg"=w983) -> ("rad"=w972:dbl)  [unwired: 9 in, 1 out]
                    n665 = feedback #18(0.0 ("Real Matrix Element")) -> (w987:dbl)
                    n666 = feedback-in #18(w988) -> ()
                    n667 = feedback #19(0.0 ("Real Matrix Element")) -> (w986:dbl)
                    n668 = feedback-in #19(w985) -> ()
                    n669 = Not Equal?(x=w988, y=w987) -> (x != y?=w994:bool)
                    n670 = Not Equal?(x=w985, y=w986) -> (x != y?=w979:bool)
                    n671 = Not Equal To 0?(x=w993) -> (x != 0?=w992:bool)
                    n672 = Greater Or Equal To 0?(x=w1002) -> (x >= 0?=w1003:bool)
                    n673 = Absolute Value(x=w955) -> (abs(x)=w954:dbl)
                    n674 = Multiply(x=w960, y=0.5) -> (x*y=w969:dbl)
                    n675 = call "headingweightsum.vi"("a"=0.5, "h1"=w972, "h2"=w973) -> ("a*h2+(1-a)*h1"=w1001:dbl)  [unwired: 8 in]
                    n676 = And(x=w994, y=w992) -> (x .and. y?=w975:bool)
                    n677 = And(x=w979, y=w981) -> (x .and. y?=w974:bool)
                    n678 = Divide(x=w969, y=w954) -> (x/y=w970:dbl)
                    n679 = Select(t=0.0, s=w1003, f=3.141592653589793) -> (s? t:f=w1000:dbl)
                    n680 = call "headingoperater.vi"("h1"=w1000, "h2"=w1001) -> ("h2-h1"=w999:dbl)  [unwired: 8 in, 1 out]
                    n681 = Decrement(x=w970) -> (x-1=w966:dbl)
                    n682 = Absolute Value(x=w966) -> (abs(x)=w967:dbl)
                    n683 = And(x=w975, y=w974) -> (x .and. y?=w998:bool)
                    n684 = Greater?(x=w954, y=15.0) -> (0:w956:bool)
                    n685 = Less?(x=w967, y=0.05) -> (x < y?=w959:bool)
                    n686 = Compound Arithmetic op=AND(w956, w959, w998) -> (w958:bool)
                  }
                  frame Enabled {
                    n687 = global read "rio_Global.vi" "gps_vel 1"() -> (w1029:dbl[])
                    n688 = global read "rio_Global.vi" "C_VS_CAN"() -> (w1006:dbl)
                    n689 = Index Array(array=w1029, index #1=2 ("index"), index #2=4 ("index"), index #3=0 ("index"), index #4=1 ("index")) -> (element #1=w1009:dbl, element #2=w1007:dbl, element #3=w1014:dbl, element #4=w1025:dbl)
                    n690 = Greater Or Equal To 0?(x=w1006) -> (x >= 0?=w1032:bool)
                    n691 = Absolute Value(x=w1006) -> (abs(x)=w1016:dbl)
                    n692 = feedback #20(w1014) -> (w1023:dbl)
                    n693 = feedback-in #20(w1014) -> ()
                    n694 = Divide(x=w1009, y=w1016) -> (x/y=w1022:dbl)
                    n695 = call "angleconv.vi"("deg"=w1007) -> ("rad"=w1015:dbl)  [unwired: 9 in, 1 out]
                    n696 = Select(t=0.0, s=w1032, f=3.141592653589793) -> (s? t:f=w1031:dbl)
                    n697 = Not Equal?(x=w1014, y=w1023) -> (x != y?=w1026:bool)
                    n698 = call "headingoperater.vi"("h1"=w1031, "h2"=w1015) -> ("h2-h1"=w1030:dbl)  [unwired: 8 in, 1 out]
                    n699 = Decrement(x=w1022) -> (x-1=w1019:dbl)
                    n700 = Not Equal To 0?(x=w1025) -> (x != 0?=w1024:bool)
                    n701 = Absolute Value(x=w1019) -> (abs(x)=w1020:dbl)
                    n702 = And(x=w1026, y=w1024) -> (x .and. y?=w1011:bool)
                    n703 = Greater?(x=w1016, y=15.0) -> (0:w1012:bool)
                    n704 = Less?(x=w1020, y=0.2) -> (x < y?=w1013:bool)
                    n705 = Compound Arithmetic op=AND(w1013, w1012, w1011) -> (w1018:bool)
                  }
                }
                n706 = disable-structure shown="Enabled" {
                  disable-tunnel: [w928 w937] -> w896
                  disable-tunnel: [w909 w947] -> w895
                  disable-tunnel: [_ w929] -> w893
                  frame Disabled {
                    n707 = global read "rio_Global.vi" "gps_pos 1"() -> (w925:dbl[])
                    n708 = global read "rio_Global.vi" "gps_pos 2"() -> (w912:dbl[])
                    n709 = Add(x=w925, y=w912) -> (x+y=w927:dbl[])
                    n710 = Index Array(array=w925, index #1=0 ("index")) -> (element #1=w924:dbl, element #2=w923:dbl)  [unwired: 1 in]
                    n711 = Index Array(array=w912, index #1=0 ("index")) -> (element #1=w913:dbl, element #2=w914:dbl)  [unwired: 1 in]
                    n712 = feedback #21(w924) -> (w922:dbl)
                    n713 = feedback-in #21(w924) -> ()
                    n714 = feedback #22(w913) -> (w915:dbl)
                    n715 = feedback-in #22(w913) -> ()
                    n716 = Not Equal?(x=w924, y=w922) -> (x != y?=w921:bool)
                    n717 = Not Equal?(x=w913, y=w915) -> (x != y?=w916:bool)
                    n718 = Not Equal To 0?(x=w923) -> (x != 0?=w920:bool)
                    n719 = Not Equal To 0?(x=w914) -> (x != 0?=w917:bool)
                    n720 = And(x=w921, y=w920) -> (x .and. y?=w910:bool)
                    n721 = And(x=w916, y=w917) -> (x .and. y?=w911:bool)
                    n722 = And(x=w910, y=w911) -> (x .and. y?=w928:bool)
                    n723 = Multiply(x=w927, y=0.5) -> (x*y=w909:dbl[])
                  }
                  frame Enabled {
                    w931 = 250 ("x")
                    n724 = global read "rio_Global.vi" "gps_pos 1"() -> (w947:dbl[])
                    n725 = Index Array(array=w947, index #1=0 ("index"), index #3=6 ("index"), index #4=9 ("index")) -> (element #1=w953:dbl, element #2=w952:dbl, element #3=w944:dbl, element #4=w942:dbl)  [unwired: 1 in]
                    n726 = local read "conutpos"() -> (w935:i32)
                    n727 = feedback #23(w953) -> (w951:dbl)
                    n728 = feedback-in #23(w953) -> ()
                    n729 = Greater?(x=w944, y=10.0) -> (0:w940:bool)
                    n730 = Less?(x=w942, y=1.5) -> (x < y?=w939:bool)
                    n731 = Not Equal?(x=w953, y=w951) -> (x != y?=w950:bool)
                    n732 = And(x=w940, y=w939) -> (x .and. y?=w936:bool)
                    n733 = Not Equal To 0?(x=w952) -> (x != 0?=w949:bool)
                    n734 = Increment(x=w935) -> (x+1=w934:i32)
                    n735 = And(x=w950, y=w949) -> (x .and. y?=w938:bool)
                    n736 = Select(t=w934, s=w936, f=0) -> (s? t:f=w932:i32)
                    n737 = Max & Min(x=w931, y=w932) -> (min(x,y)=w930:i32)  [unwired: 1 out]
                    n738 = local write "conutpos"(w930) -> ()
                    n739 = Equal?(x=w931, y=w930) -> (x = y?=w929:bool)
                    n740 = And(x=w938, y=w929) -> (x .and. y?=w937:bool)
                  }
                }
                "pos_gps" <- w895
                n741 = local write "h_gps"(w898) -> ()
                n742 = local write "get position"(w896) -> ()
                n743 = case shown="True" w890 {
                  tunnel: w897 -> [_ w1042]
                  frame False {
                  }
                  frame True {
                    w1036 = u64 18446744073709551615
                    n744 = local read "vcount"() -> (w1039:u64)
                    n745 = local read "vgain"() -> (w1044:dbl)
                    n746 = Increment(x=w1039) -> (x+1=w1038:u64)
                    n747 = Not Equal?(x=w1039, y=w1036) -> (x != y?=w1037:bool)
                    n748 = Multiply(x=w1044, y=w1039) -> (x*y=w1043:dbl)
                    n749 = Add(x=w1042, y=w1043) -> (x+y=w1041:dbl)
                    n750 = Select(t=w1038, s=w1037, f=w1036) -> (s? t:f=w1035:u64)
                    n751 = local write "vcount"(w1035) -> ()
                    n752 = Divide(x=w1041, y=w1035) -> (x/y=w1040:dbl)
                    n753 = local write "vgain"(w1040) -> ()
                  }
                }
                n754 = And(x=w893, y=w894) -> (x .and. y?=w892:bool)
                n755 = Equal To 0?(x=w888) -> (x = 0?=w889:bool)
                n756 = local write "get heading"(w892) -> ()
                n757 = case shown="True" w889 {
                  frame False {
                  }
                  frame True {
                    w902 = u64 18446744073709551615
                    n758 = local read "hcount"() -> (w905:u64)
                    n759 = local read "hbias"() -> (w908:dbl)
                    n760 = Increment(x=w905) -> (x+1=w904:u64)
                    n761 = local read "C_yaw_rate"() -> (w899:dbl)
                    n762 = Not Equal?(x=w905, y=w902) -> (x != y?=w903:bool)
                    n763 = Multiply(x=w908, y=w905) -> (x*y=w907:dbl)
                    n764 = Add(x=w899, y=w907) -> (x+y=w906:dbl)
                    n765 = Select(t=w904, s=w903, f=w902) -> (s? t:f=w901:u64)
                    n766 = local write "hcount"(w901) -> ()
                    n767 = Divide(x=w906, y=w901) -> (x/y=w900:dbl)
                    n768 = local write "hbias"(w900) -> ()
                  }
                }
              }
              frame #1 {
                n769 = flat-sequence {
                  tunnel: w1047 -> [w1087]
                  tunnel: [w1066] -> w1045
                  tunnel: [w1101] -> w1046
                  tunnel: w1045 -> [w1100]
                  frame #0 {
                    n770 = local read "C_yaw_rate"() -> (w1049:dbl)
                    n771 = local read "vel_ave"() -> (w1058:dbl)
                    n772 = local read "hbias"() -> (w1057:dbl)
                    n773 = local read "vgain"() -> (w1062:dbl)
                    n774 = Subtract(x=w1049, y=w1057) -> (x-y=w1056:dbl)
                    n775 = global read "rio_Global.vi" "C_VS_CAN"() -> (w1054:dbl)
                    n776 = Multiply(x=w1058, y=w1062) -> (x*y=w1061:dbl)
                    n777 = Negate(x=w1056) -> (-x=w1055:dbl)
                    n778 = Equal To 0?(x=w1054) -> (x = 0?=w1053:bool)
                    n779 = call "angleconv.vi"("deg"=w1055) -> ("rad"=w1051:dbl)  [unwired: 9 in, 1 out]
                    n780 = Divide(x=w1061, y=3.6) -> (x/y=w1060:dbl)
                    n781 = Index Array(array=w1087, index #1=0 ("index"), index #2=3 ("index"), index #3=1 ("index"), index #4=3 ("index")) -> (element #1=w1081:dbl, element #2=w1079:dbl, element #3=w1075:dbl, element #4=w1070:dbl)
                    n782 = local read "dt vel"() -> (w1084:dbl)
                    n783 = Select(t=0.0, s=w1053, f=w1051) -> (s? t:f=w1050:dbl)
                    n784 = local read "dt yaw"() -> (w1059:dbl)
                    n785 = Cosine(x=w1079) -> (cos(x)=w1085:dbl)
                    n786 = Multiply(x=w1060, y=w1084) -> (x*y=w1080:dbl)
                    n787 = Sine(x=w1079) -> (sin(x)=w1078:dbl)
                    n788 = Multiply(x=w1085, y=w1080) -> (x*y=w1082:dbl)
                    n789 = Multiply(x=w1080, y=w1078) -> (x*y=w1077:dbl)
                    n790 = Multiply(x=w1059, y=w1050) -> (x*y=w1048:dbl)
                    n791 = Add(x=w1081, y=w1082) -> (x+y=w1074:dbl)
                    n792 = Add(x=w1077, y=w1075) -> (x+y=w1073:dbl)
                    n793 = call "headingoperater.vi"("h1"=w1048, "h2"=w1070) -> ("h2+h1"=w1069:dbl)  [unwired: 8 in, 1 out]
                    n794 = Build Array(w1074, w1073, w1060, w1069, w1050) -> (w1066:dbl[])
                    n795 = Index Array(array=w1066, index=3) -> (element=w1065:dbl)
                    n796 = local read "h_gps"() -> (w1064:dbl)
                    n797 = call "headingoperater.vi"("h1"=w1065, "h2"=w1064) -> ("h2-h1"=w1068:dbl)  [unwired: 8 in, 1 out]
                    n798 = Absolute Value(x=w1068) -> (abs(x)=w1063:dbl)
                    n799 = local write "heading error"(w1063) -> ()
                  }
                  frame #1 {
                    n800 = global read "rio_Global.vi" "C_VS_CAN"() -> (w1106:dbl)
                    n801 = local read "heading error"() -> (w1096:dbl)
                    n802 = Absolute Value(x=w1106) -> (abs(x)=w1105:dbl)
                    n803 = local read "get heading"() -> (w1108:bool)
                    n804 = local read "get position"() -> (w1107:bool)
                    n805 = local read "POS init"() -> (w1094:bool)
                    n806 = Or(x=w1108, y=w1107) -> (x .or. y?=w1103:bool)
                    n807 = Greater?(x=w1105, y="GPS Update km/h") -> (0:w1102:bool)
                    n808 = Less?(x=w1096, y=1.0) -> (x < y?=w1095:bool)
                    n809 = Or(x=w1095, y=w1094) -> (x .or. y?=w1097:bool)
                    n810 = And(x=w1103, y=w1102) -> (x .and. y?=w1098:bool)
                    n811 = And(x=w1098, y=w1097) -> (x .and. y?=w1090:bool)
                    n812 = Select(t=w1090, s="GPS on", f="GPS on") -> (s? t:f=w1089:bool)
                    n813 = Select(t=FALSE, s="GPS init", f=w1089) -> (s? t:f=w1092:bool)
                    n814 = case shown="True" w1092 {
                      tunnel: [w1112 w1141] -> w1101
                      tunnel: w1100 -> [w1113 w1144]
                      frame False {
                        n815 = global read "rio_Global.vi" "C_VS_CAN"() -> (w1116:dbl)
                        n816 = local read "POS init"() -> (w1115:bool)
                        n817 = Equal To 0?(x=w1116) -> (x = 0?=w1114:bool)
                        n818 = local read "GPS init"() -> (w1109:bool)
                        n819 = And(x=w1115, y=w1114) -> (x .and. y?=w1111:bool)
                        n820 = Or(x=w1111, y=w1109) -> (x .or. y?=w1110:bool)
                        n821 = case shown="False" w1110 {
                          tunnel: w1113 -> [w1117 w1118]
                          tunnel: [w1117 w1120] -> w1112
                          tunnel: w1109 -> [_ w1119]
                          frame False {
                          }
                          frame True {
                            n822 = case shown="False" w1119 {
                              tunnel: [w1131 w1140] -> w1120
                              tunnel: w1118 -> [w1126 w1134]
                              frame True {
                                n823 = Index Array(array=w1126, index #1=2 ("index")) -> (element #2=w1121:dbl, element #3=w1124:dbl)  [unwired: 2 in, 1 out]
                                n824 = local read "pos_gps"() -> (w1127:dbl[])
                                n825 = local write "GPS init"(FALSE ("GPS init")) -> ()
                                n826 = Index Array(array=w1127, index #1=2 ("index")) -> (element #1=w1129:dbl, element #2=w1128:dbl)  [unwired: 1 in]
                                n827 = local read "h_gps"() -> (w1122:dbl)
                                n828 = Build Array(w1129, w1128, w1121, w1122, w1124) -> (w1131:dbl[])
                              }
                              frame False {
                                w1133 = 0.0 ("element")
                                n829 = Index Array(array=w1134, index=3) -> (element=w1132:dbl)
                                n830 = local read "pos_gps"() -> (w1136:dbl[])
                                n831 = Index Array(array=w1136, index #1=2 ("index")) -> (element #1=w1138:dbl, element #2=w1137:dbl)  [unwired: 1 in]
                                n832 = Build Array(w1138, w1137, w1133, w1132, w1133) -> (w1140:dbl[])
                              }
                            }
                          }
                        }
                      }
                      frame True {
                        n833 = flat-sequence {
                          tunnel: w1144 -> [w1145]
                          tunnel: [w1145] -> w1143
                          tunnel: w1143 -> [w1186]
                          tunnel: [w1186] -> w1142
                          tunnel: w1142 -> [w1224]
                          tunnel: [w1228] -> w1141
                          frame #0 {
                            w1154 = 0.0 ("element")
                            w1158 = 0.0 ("element")
                            w1160 = 0.0 ("element")
                            w1162 = 0.0 ("element")
                            w1164 = 0.0 ("element")
                            n834 = Index Array(array=w1145, index #1=3 ("index"), index #2=2 ("index"), index #3=3 ("index"), index #4=2 ("index")) -> (element #1=w1174:dbl, element #2=w1176:dbl, element #3=w1179:dbl, element #4=w1168:dbl)
                            n835 = Negate(x=w1176) -> (-x=w1175:dbl)
                            n836 = Sine & Cosine(0:w1179) -> (1:w1171:dbl, 2:w1169:dbl)
                            n837 = Multiply(x=w1175, y=w1171) -> (x*y=w1172:dbl)
                            n838 = Multiply(x=w1169, y=w1168) -> (x*y=w1167:dbl)
                            n839 = Cosine(x=w1174) -> (cos(x)=w1173:dbl)
                            n840 = Build Array(w1164, w1164, w1173, w1172, 0.0 ("element")) -> (w1166:dbl[])
                            n841 = Build Array(w1162, w1162, w1171, w1167, 0.0 ("element")) -> (w1165:dbl[])
                            n842 = Build Array(w1160, w1160, w1160, w1160, w1160) -> (w1159:dbl[])
                            n843 = Build Array(w1158, w1158, w1158, w1158, 1.0 ("element")) -> (w1156:dbl[])
                            n844 = Build Array(w1154, w1154, w1154, w1154, w1154) -> (w1155:dbl[])
                            n845 = Build Array(w1166, w1165, w1159, w1156, w1155) -> (w1152:dbl[][])
                            n846 = call-poly <vilib>:"Array To Matrix.vi"("Real 2D Array"=w1152) -> ("Real Matrix"=w1150:T19)
                            n847 = global read "rio_Global.vi" "P"() -> (w1153:T19)
                            n848 = Transpose Matrix(1:w1150) -> (0:w1149:T19)
                            n849 = call-poly <vilib>:"Multiply.vi"("Real Matrix B"=w1153, "Real Matrix A"=w1150) -> ("A * B"=w1151:T19)
                            n850 = call-poly <vilib>:"Multiply.vi"("Real Matrix B"=w1149, "Real Matrix A"=w1151) -> ("A * B"=w1148:T19)
                            n851 = global read "rio_Global.vi" "Q"() -> (w1147:T19)
                            n852 = call-poly <vilib>:"Add.vi"("Real Matrix B"=w1147, "Real Matrix A"=w1148) -> ("A + B"=w1146:T19)
                            n853 = global write "rio_Global.vi" "Pp"(w1146) -> ()
                          }
                          frame #1 {
                            n854 = global read "rio_Global.vi" "Pp"() -> (w1211:T19)
                            n855 = global read "rio_Global.vi" "H"() -> (w1210:T19)
                            n856 = Array Subset(array=w1186, index=0, length=2) -> (w1193:dbl[])
                            n857 = local read "pos_gps"() -> (w1189:dbl[])
                            n858 = call-poly <vilib>:"Multiply.vi"("Real Matrix B"=w1211, "Real Matrix A"=w1210) -> ("A * B"=w1209:T19)
                            n859 = Transpose Matrix(1:w1210) -> (0:w1208:T19)
                            n860 = call-poly <vilib>:"Multiply.vi"("Real Matrix B"=w1208, "Real Matrix A"=w1209) -> ("A * B"=w1207:T19)
                            n861 = Array Subset(array=w1189, index=2, length=2) -> (w1192:dbl[])
                            n862 = Subtract(x=w1192, y=w1193) -> (x-y=w1194:dbl[])
                            n863 = global read "rio_Global.vi" "H"() -> (w1205:T19)
                            n864 = global read "rio_Global.vi" "R"() -> (w1206:T19)
                            n865 = global read "rio_Global.vi" "Pp"() -> (w1204:T19)
                            n866 = call-poly <vilib>:"Add.vi"("Real Matrix B"=w1206, "Real Matrix A"=w1207) -> ("A + B"=w1201:T19)
                            n867 = Square(x=w1194) -> (x^2=w1195:dbl[])
                            n868 = Transpose Matrix(1:w1205) -> (0:w1203:T19)
                            n869 = local read "heading error"() -> (w1198:dbl)
                            n870 = call-poly <vilib>:"Multiply.vi"("Real Matrix B"=w1203, "Real Matrix A"=w1204) -> ("A * B"=w1202:T19)
                            n871 = Add Array Elements(numeric array=w1195) -> (sum=w1196:dbl)
                            n872 = call-poly <vilib>:"Inverse Matrix.vi"("Input Matrix"=w1201) -> ("Inverse Matrix"=w1200:T19)  [unwired: 1 in, 1 out]
                            n873 = call-poly <vilib>:"Multiply.vi"("Real Matrix B"=w1200, "Real Matrix A"=w1202) -> ("A * B"=w1199:T19)
                            n874 = Square Root(x=w1196) -> (sqrt(x)=w1181:dbl)
                            n875 = global write "rio_Global.vi" "K"(w1199) -> ()
                            n876 = local write "pos error"(w1181) -> ()
                            n877 = Less?(x=w1181, y=2.5) -> (x < y?=w1183:bool)
                            n878 = Less?(x=w1198, y=0.05) -> (x < y?=w1184:bool)
                            n879 = And(x=w1184, y=w1183) -> (x .and. y?=w1182:bool)
                            n880 = case shown="True" w1182 {
                              frame False {
                              }
                              frame True {
                                n881 = local write "POS init"(FALSE ("Kalman init")) -> ()
                              }
                            }
                          }
                          frame #2 {
                            n882 = Index Array(array=w1224, index=3) -> (element=w1231:dbl)
                            n883 = global read "rio_Global.vi" "K"() -> (w1239:T19)
                            n884 = global read "rio_Global.vi" "H"() -> (w1238:T19)
                            n885 = local read "heading error"() -> (w1219:dbl)
                            n886 = global read "rio_Global.vi" "Pp"() -> (w1236:T19)
                            n887 = call-poly <vilib>:"Multiply.vi"("Real Matrix B"=w1238, "Real Matrix A"=w1239) -> ("A * B"=w1237:T19)
                            n888 = local read "pos error"() -> (w1220:dbl)
                            n889 = global read "rio_Global.vi" "Pp"() -> (w1234:T19)
                            n890 = call-poly <vilib>:"Multiply.vi"("Real Matrix B"=w1236, "Real Matrix A"=w1237) -> ("A * B"=w1235:T19)
                            n891 = local read "get position"() -> (w1222:bool)
                            n892 = local read "get heading"() -> (w1216:bool)
                            n893 = call-poly <vilib>:"Subtract.vi"("Real Matrix B"=w1235, "Real Matrix A"=w1234) -> ("A - B"=w1233:T19)
                            n894 = Greater?(x=50.0, y=w1220) -> (0:w1221:bool)
                            n895 = Less?(x=w1219, y=0.1 ("y 2")) -> (x < y?=w1217:bool)
                            n896 = local read "POS init"() -> (w1213:bool)
                            n897 = global write "rio_Global.vi" "P"(w1233) -> ()
                            n898 = And(x=w1222, y=w1221) -> (x .and. y?=w1215:bool)
                            n899 = And(x=w1216, y=w1217) -> (x .and. y?=w1214:bool)
                            n900 = Or(x=w1215, y=w1213) -> (x .or. y?=w1226:bool)
                            n901 = Or(x=w1213, y=w1214) -> (x .or. y?=w1227:bool)
                            n902 = case shown="True" w1227 {
                              tunnel: w1231 -> [w1261 w1268]
                              tunnel: [w1261 w1267] -> w1225
                              frame False {
                              }
                              frame True {
                                n903 = global read "rio_Global.vi" "K"() -> (w1266:T19)
                                n904 = Index Array(array=w1266, index (row)=3, index (col)=2 ("disabled index (col)")) -> (element=w1262:dbl)
                                n905 = local read "h_gps"() -> (w1263:dbl)
                                n906 = call "headingweightsum2.vi"("a"=w1262, "h2"=w1263, "h1"=w1268) -> ("a*h2+(1-a)*h1"=w1267:dbl)  [unwired: 8 in]
                              }
                            }
                            n907 = case shown="True" w1226 {
                              tunnel: w1224 -> [w1240 w1251]
                              tunnel: [w1240 w1250] -> w1230
                              tunnel: w1225 -> [_ w1242]
                              frame False {
                              }
                              frame True {
                                n908 = local read "pos_gps"() -> (w1246:dbl[])
                                n909 = call-poly <vilib>:"Array To Matrix.vi"("Real 1D Array"=w1251) -> ("Real Matrix (Column Vector)"=w1255:T19)
                                n910 = Array Subset(array=w1246, index=2, length=2) -> (w1247:dbl[])
                                n911 = Build Array (concatenate)(w1247, w1242) -> (w1243:dbl[])
                                n912 = global read "rio_Global.vi" "H"() -> (w1260:T19)
                                n913 = call-poly <vilib>:"Multiply.vi"("Real Matrix B"=w1255, "Real Matrix A"=w1260) -> ("A * B"=w1259:T19)
                                n914 = call-poly <vilib>:"Array To Matrix.vi"("Real 1D Array"=w1243) -> ("Real Matrix (Column Vector)"=w1258:T19)
                                n915 = call-poly <vilib>:"Subtract.vi"("Real Matrix B"=w1259, "Real Matrix A"=w1258) -> ("A - B"=w1256:T19)
                                n916 = global read "rio_Global.vi" "K"() -> (w1257:T19)
                                n917 = call-poly <vilib>:"Multiply.vi"("Real Matrix B"=w1256, "Real Matrix A"=w1257) -> ("A * B"=w1241:T19)
                                n918 = call-poly <vilib>:"Multiply.vi"("Real Matrix A"=w1241, "Real Scalar c"=0.5) -> ("c * A"=w1248:T19)
                                n919 = call-poly <vilib>:"Add.vi"("Real Matrix B"=w1255, "Real Matrix A"=w1248) -> ("A + B"=w1254:T19)
                                n920 = call-poly <vilib>:"Matrix To Array.vi"("Real Matrix"=w1254) -> ("Real 2D Array"=w1253:dbl[][])
                                n921 = Index Array(array=w1253, index (col)=0 ("disabled index (col)")) -> (element=w1250:dbl[])  [unwired: 1 in]
                              }
                            }
                            n922 = Replace Array Subset(array=w1230, new element=w1225, index=3) -> (w1228:dbl[])
                          }
                        }
                      }
                    }
                  }
                }
              }
            }
          }
          frame #2 {
            n923 = local read "dt yaw"() -> (w1271:dbl)
            n924 = local read "h_gps"() -> (w1274:dbl)
            n925 = Index Array(array=w1285, index=3) -> (element=w1278:dbl)
            n926 = Array Subset(array=w1285, index=0, length=2) -> (→"pos":dbl[])
            n927 = Greater Than 0?(x=w1271) -> (x > 0?=w1270:bool)
            n928 = call "angleconv.vi"("rad"=w1278) -> ("deg"=→"Heading":dbl)  [unwired: 9 in, 1 out]
            n929 = Greater?(x=1.0, y=w1271) -> (0:w1273:bool)
            n930 = call "headingoperater.vi"("h1"=0.0, "h2"=w1274) -> ("h2+h1"=w1275:dbl)  [unwired: 8 in, 1 out]
            n931 = call "angleconv.vi"("rad"=w1275) -> ("deg"=→"H_GPS":dbl)  [unwired: 9 in, 1 out]
            n932 = Compound Arithmetic op=AND(w1273, w1270) -> (w1269:bool)
            n933 = case shown="True" w1269 {
              tunnel: w1285 -> [_ w1286]
              frame False {
              }
              frame True {
                n934 = flat-sequence {
                  tunnel: w1286 -> [w1310]
                  frame #0 {
                    n935 = Get Date/Time In Seconds() -> (seconds since 1Jan1904=w1301:timestamp)
                    n936 = To Double Precision Float(number=w1301) -> (double precision float=w1295:dbl)
                    n937 = global read "rio_Global.vi" "LCM_POS_T"() -> (w1309:T20)
                    n938 = local read "POS init"() -> (w1291:bool)
                    n939 = local read "dt yaw"() -> (w1290:dbl)
                    n940 = Unbundle By Name(w1309) -> ("hash"=w1306:i64)
                    n941 = Multiply(x=w1295, y=1000000.0) -> (x*y=w1293:dbl)
                    n942 = Array To Cluster(array=w1310) -> (cluster=w1308:T21)
                    n943 = To Quad Integer(1:w1293) -> (0:w1292:i64)
                    n944 = call "hash.vi"("input"=w1306) -> ("output"=w1305:i64)  [unwired: 10 in]
                    n945 = Unbundle(w1308) -> ("Real 2D Array[0]"=w1300:dbl, "Real 2D Array[1]"=w1299:dbl, "Real 2D Array[2]"=w1298:dbl, "Real 2D Array[3]"=w1297:dbl, "Real 2D Array[4]"=w1296:dbl)
                    n946 = Select(t=0.0, s=w1291, f=w1290) -> (s? t:f=w1288:dbl)
                    n947 = Bundle(cluster=w1309, "hash"=w1305, "sys time"=w1292, "dt"=w1288, "x"=w1300, "y"=w1299, "speed"=w1298, "heading"=w1297, "yaw_rate"=w1296) -> (w1287:T20)
                    n948 = Flatten To String(anything=w1287, prepend array or string size? (T)=FALSE) -> (data string=w1303:string)  [unwired: 2 in, 2 out]
                    n949 = global read "rio_Global.vi" "LCM"() -> (w1302:T4)
                    n950 = call "LCM_send.vi"("DATA"=w1303, "ID"="POS_T", "LCM"=w1302) -> ()  [unwired: 7 in, 2 out]
                  }
                }
              }
            }
          }
        }
        n951 = node-c288() -> ()  [unwired: 1 in, 1 out]
      }
      n952 = node-c288(w839) -> ()  [unwired: 1 out]
    }
  }
